vi "eventMode.vi"() -> ()   [LabVIEW 2019]
uses:
  TypeDefs/pixArrSmol.ctl
  <vilib>/Math Plots/3D Math Plots/3D Surface/3D Surface XCtrl/3D Surface.xctl
  <vilib>/Utility/error.llb/whitespace.ctl
  <vilib>/Instr/_visa.llb/VISA Flush IO Buffer Mask.ctl
  <vilib>/Utility/file.llb/Read Delimited Spreadsheet (string).vi
  <vilib>/Math Plots/3D Math Plots/3D Surface/3D Surface Datatype/Public/Plot Helper (Vector).vi
  <vilib>/Instr/_visa.llb/VISA Configure Serial Port (Instr).vi
  TypeDefs/serialSettings_Global.vi
  <vilib>/Analysis/NI_AALBase.lvlib
  <vilib>/Math Plots/3D Math Plots/3D Surface/3D Surface Datatype/3D Surface Datatype.lvclass
panel:
  out "read buffer":string
  out "Noisy Pixel List":i32[][](array[numeric])
  out "all rows":string[][](array[string])
  in  "Open CSV":bool
  out "Intensity Graph":u32[][](graph)
  out "States Out":string
  out "Current Time":timestamp
  in  "Iteration Limit":u32=4999
  out "Detector Surface":refnum<class "3D Plot Datatype.lvclass">[](xcontrol)
  out "Event Count Histogram":T1(graph)
  in  "Set emulate":bool
  out "Emulator 1":bool
  in  "Emulate?":bool
  out "Emulator 2":bool
  out "CZT 2 \nFrequency":u8 format="%d Mhz"
  in  "Set Clock":bool
  in  "Set CZT Clock":u8(ring)=2 items=["30 Mhz"=6, "25 Mhz"=5, "20 Mhz"=4, "15 Mhz"=3, "10 Mhz"=2]
  out "CZT 1\nFrequency":u8 format="%d Mhz"
  in  "Detector Chooser":bool caption="Boolean"
  out "CZT 2 Threshold":u16 format="%u KeV"
  out "Serial Number 2":u32
  out "Serial Number":u32
  in  "Clear Serial":bool
  in  "Read Serial":bool
  in  "PixOff":bool
  in  "Stop":bool
  in  "Get All Pixel Status":bool
  in  "Test Description":string caption="(Inserted in FITS header)"
  out "CZT 1 Threshold":u16 format="%u KeV"
  in  "Set Threshold":bool
  in  "Select Threshold Value":u16(slide)=20 min=20 max=200 scale=20.0..200.0
  out "Column":u8=1
  out "Row":string="A"
  out "Pixel Matrix Status":T2=[[TRUE, TRUE, TRUE, TRUE, TRUE, TRUE, TRUE, TRUE, TRUE, TRUE, TRUE, TRUE, TRUE, TRUE, TRUE, TRUE, TRUE], [TRUE, TRUE, TRUE, TRUE, TRUE, TRUE, TRUE, TRUE, TRUE, TRUE, TRUE, TRUE, TRUE, TRUE, TRUE, TRUE, TRUE], [TRUE, TRUE, TRUE, TRUE, TRUE, TRUE, TRUE, TRUE, TRUE, TRUE, TRUE, TRUE, TRUE, TRUE, TRUE, TRUE, TRUE], [TRUE, TRUE, TRUE, TRUE, TRUE, TRUE, TRUE, TRUE, TRUE, TRUE, TRUE, TRUE, TRUE, TRUE, TRUE, TRUE, TRUE], [TRUE, TRUE, TRUE, TRUE, TRUE, TRUE, TRUE, TRUE, TRUE, TRUE, TRUE, TRUE, TRUE, TRUE, TRUE, TRUE, TRUE], [TRUE, TRUE, TRUE, TRUE, TRUE, TRUE, TRUE, TRUE, TRUE, TRUE, TRUE, TRUE, TRUE, TRUE, TRUE, TRUE, TRUE], [TRUE, TRUE, TRUE, TRUE, TRUE, TRUE, TRUE, TRUE, TRUE, TRUE, TRUE, TRUE, TRUE, TRUE, TRUE, TRUE, TRUE], [TRUE, TRUE, TRUE, TRUE, TRUE, TRUE, TRUE, TRUE, TRUE, TRUE, TRUE, TRUE, TRUE, TRUE, TRUE, TRUE, TRUE], [TRUE, TRUE, TRUE, TRUE, TRUE, TRUE, TRUE, TRUE, TRUE, TRUE, TRUE, TRUE, TRUE, TRUE, TRUE, TRUE, TRUE], [TRUE, TRUE, TRUE, TRUE, TRUE, TRUE, TRUE, TRUE, TRUE, TRUE, TRUE, TRUE, TRUE, TRUE, TRUE, TRUE, TRUE], [TRUE, TRUE, TRUE, TRUE, TRUE, TRUE, TRUE, TRUE, TRUE, TRUE, TRUE, TRUE, TRUE, TRUE, TRUE, TRUE, TRUE], [TRUE, TRUE, TRUE, TRUE, TRUE, TRUE, TRUE, TRUE, TRUE, TRUE, TRUE, TRUE, TRUE, TRUE, TRUE, TRUE, TRUE], [TRUE, TRUE, TRUE, TRUE, TRUE, TRUE, TRUE, TRUE, TRUE, TRUE, TRUE, TRUE, TRUE, TRUE, TRUE, TRUE, TRUE], [TRUE, TRUE, TRUE, TRUE, TRUE, TRUE, TRUE, TRUE, TRUE, TRUE, TRUE, TRUE, TRUE, TRUE, TRUE, TRUE, TRUE], [TRUE, TRUE, TRUE, TRUE, TRUE, TRUE, TRUE, TRUE, TRUE, TRUE, TRUE, TRUE, TRUE, TRUE, TRUE, TRUE, TRUE], [TRUE, TRUE, TRUE, TRUE, TRUE, TRUE, TRUE, TRUE, TRUE, TRUE, TRUE, TRUE, TRUE, TRUE, TRUE, TRUE, TRUE]]
  in  "PixOn":bool
  in  "Choose Pixel To Toggle":u8 format="%02.0f"
  in  "Stop":bool
  in  "Start":bool
  in  "Short Description":string caption="(Appended to file name)"
  in  "User Name":string
  in  "Acquisition Period":T3={"Hours"=0, "Minutes"=0, "Seconds"=10}
  out "Event Mode":bool
  out "Iteration Count":u32
  out "FITS File Generated?":bool
  out "Time elapsed":dbl format="%<%H:%M:%S>t"
  in  "Exit":bool
  # "Pixel Matrix Settings"
  # "Event Mode Test"
  # "Event Start:    A0FF55\nEvent Stop:    A00055\nEmu +Eve :    A1FF55\nThresh Set:    EXXX55\nToggle Pixel: D0XX55\nChck All Pix: DFXX55\nRead Serial:   BXXX55\nClock Set:      C00X55"
  # "Need to add stop event mode command in LV state machine!"
  # "Energy Threshold Settings"
  # "KeV"
  # "Channel"
  # "Counts"
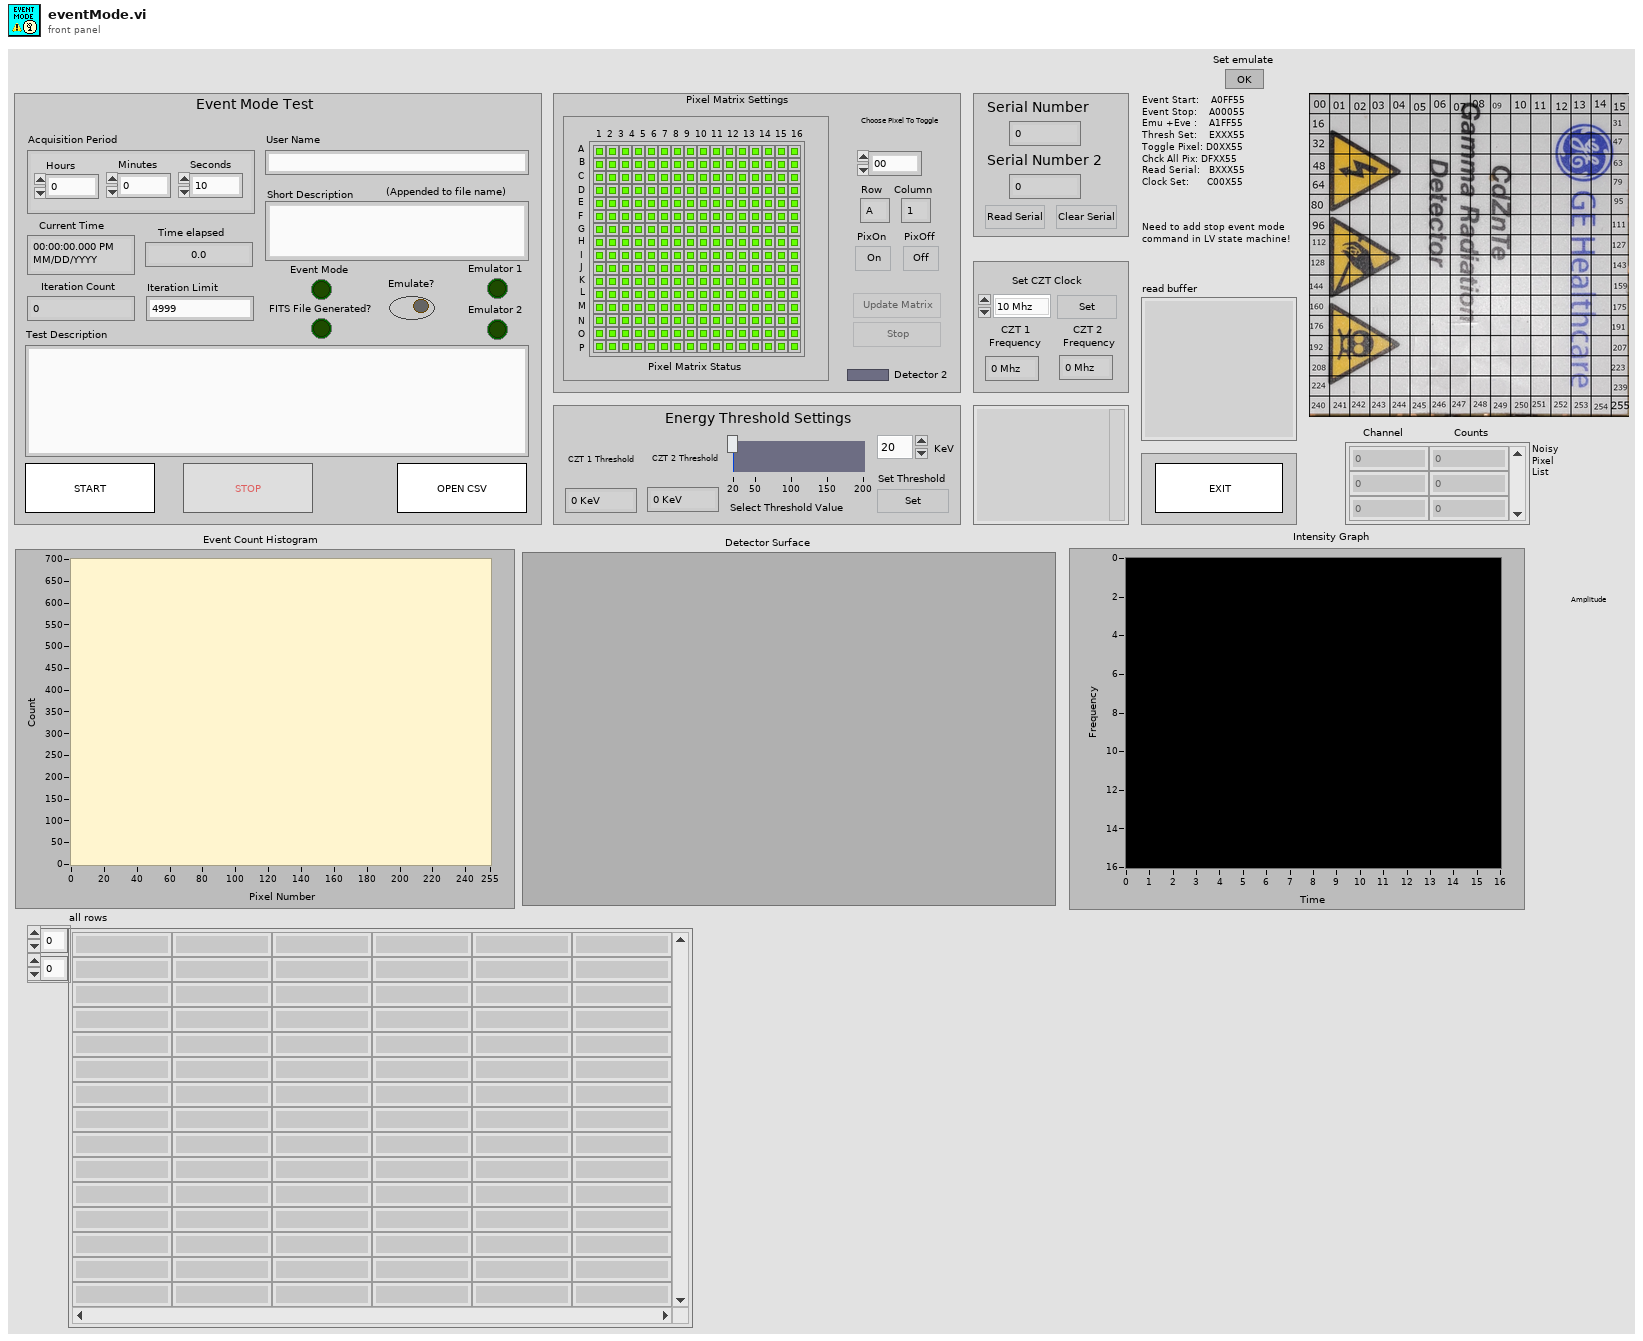
[diagram p1: front panel]
types:
  T1 = cluster{"X Values":dbl[], "Histogram: h(x)":i32[]}
  T2 = typedef "pixArrSmol.ctl" = bool[][]
  T3 = cluster{"Hours":u32, "Minutes":u32, "Seconds":u32}
  T4 = enum32{"Invalid", "Standard", "Closed", "Hidden", "Minimized", "Maximized"}
  T5 = enum32{"invalid app kind", "Development System", "Run Time System", "Student Edition", "Embedded LabVIEW", "Evaluation", "Custom"}
  T6 = enum8{"Enabled", "Disabled", "Disabled and Grayed Out"}
  T7 = cluster{"VISA resource name":refnum<visa-resource-name>, "baud rate":u32, "data bits":u16, "parity":enum16{"None", "Odd", "Even", "Mark", "Space"}, "stop bits":u16, "flow control":u16}
  T8 = cluster{"Core":cluster{"Current VI Reference":refnum<vi>, "Close Panel on Exit?":bool}, "Stop Pressed?":bool, "Start Time":dbl, "Acquisition Period":dbl, "Iteration Count":u32, "CSV File Data":cluster{"Dump txt file path":path, "Data Buffer":string, "Valid Data in Buffer":i32, "CSV file path":path, "Fits File name":string, "Test Start time":timestamp}, "User & Config Data":cluster{"User Name":string, "Short Description":string, "Description":string, "Current Threshold Value":u16}, "Pixel Status":cluster{"Pixel Number":u16, "Pixel En/Dis?":bool, "Pixel Array":bool[][], "Disabled Pixels":u8[]}}
  T9 = cluster{"Pixel Number":u16, "Pixel En/Dis?":bool, "Pixel Array":bool[][], "Disabled Pixels":u8[]}
  T10 = cluster{"User Name":string, "Short Description":string, "Description":string, "Current Threshold Value":u16}
  T11 = cluster{"Dump txt file path":path, "Data Buffer":string, "Valid Data in Buffer":i32, "CSV file path":path, "Fits File name":string, "Test Start time":timestamp}
  T12 = cluster{"Current VI Reference":refnum<vi>, "Close Panel on Exit?":bool}
  T13 = cluster{"User Name":string, "Short Description ":string, "Test Description":string, "Value":u16}
  T14 = cluster{"Dump txt file path":path, "Data buffer OUT":string, "Valid Data Buf OUT":i32, "CSV file path":path, "Fits File name":string, "Test Start time":timestamp}
  T15 = cluster{"Fits File name":string, "User Name":string, "Short Description":string, "Description":string, "Test Start time":timestamp, "Acquisition Period":dbl, "Current Threshold Value":u16, "Disabled Pixels":u8[]}
  T16 = typedef "whitespace.ctl" = u16
  T17 = typedef "VISA Flush IO Buffer Mask.ctl" = u16
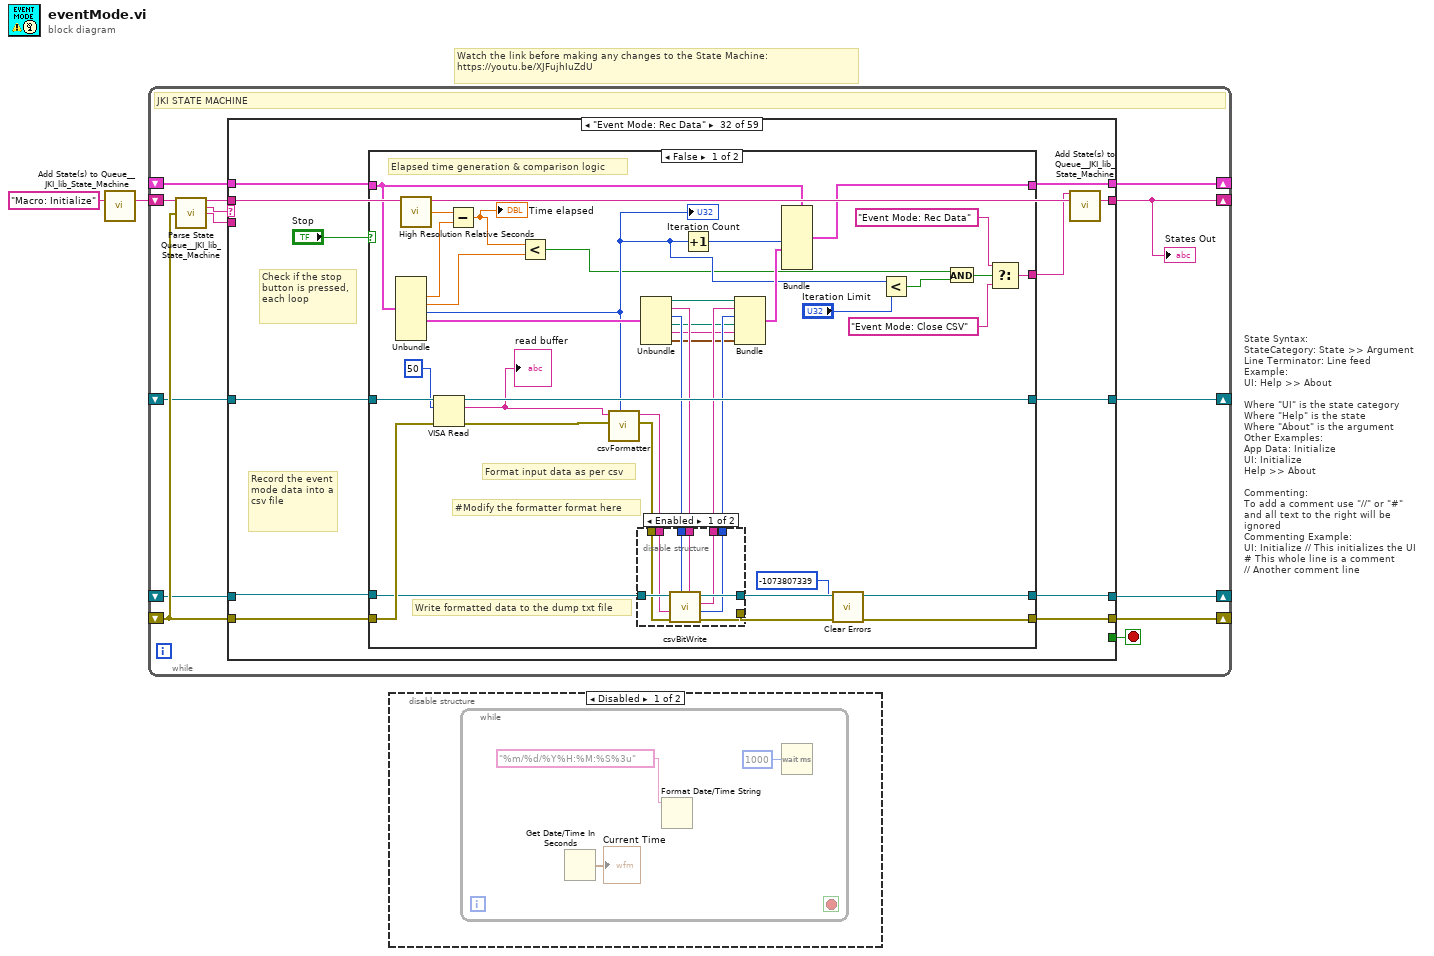
[diagram p0: block diagram]
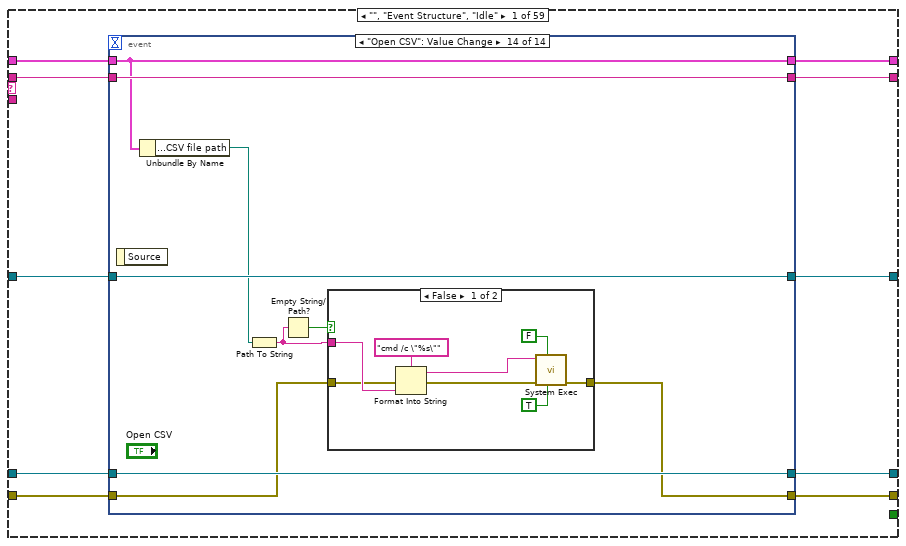
[diagram p3: hidden frame]
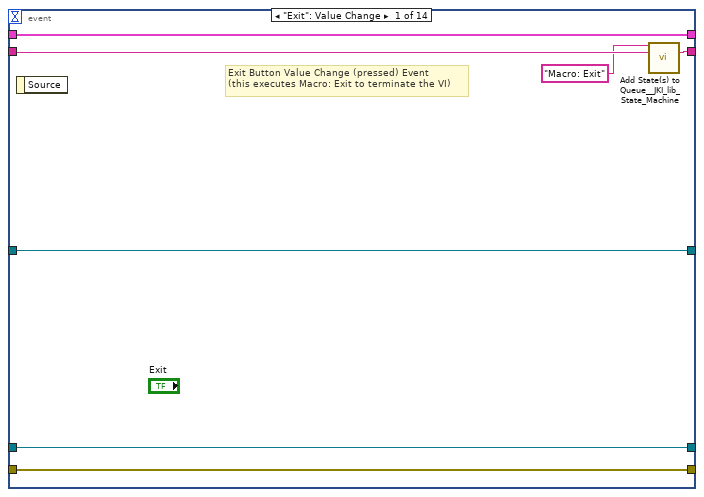
[diagram p4: hidden frame]
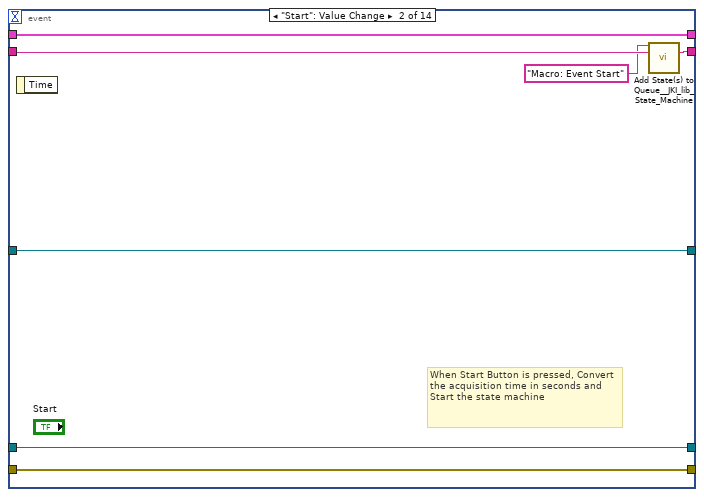
[diagram p5: hidden frame]
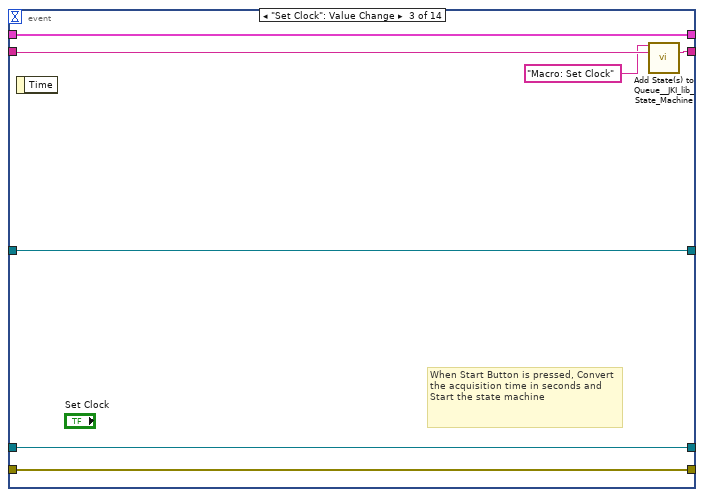
[diagram p6: hidden frame]
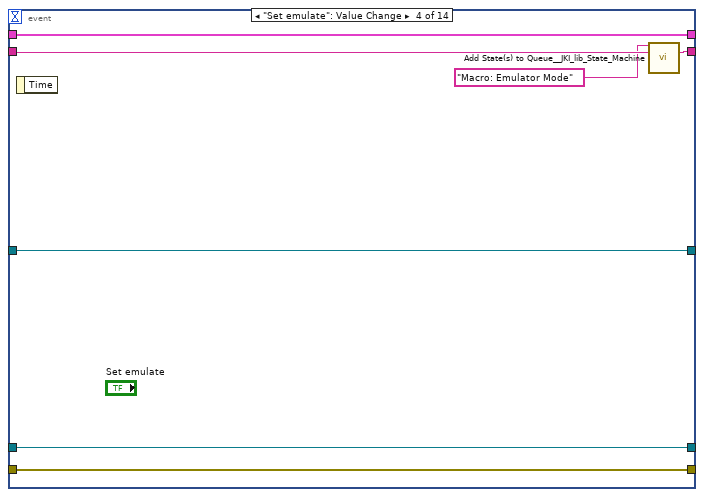
[diagram p7: hidden frame]
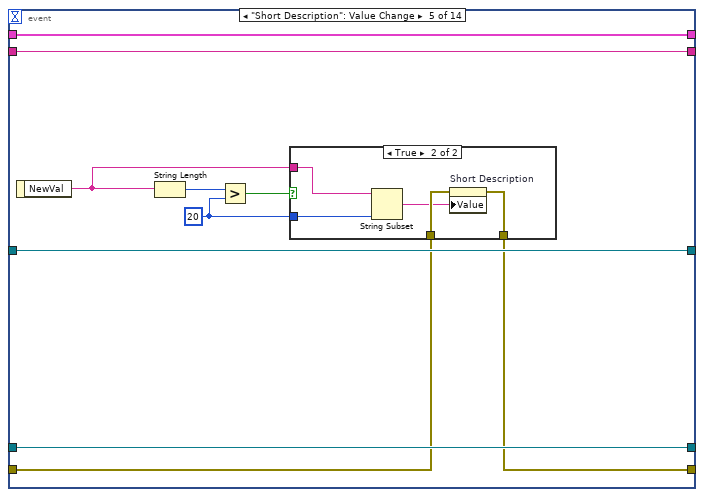
[diagram p8: hidden frame]
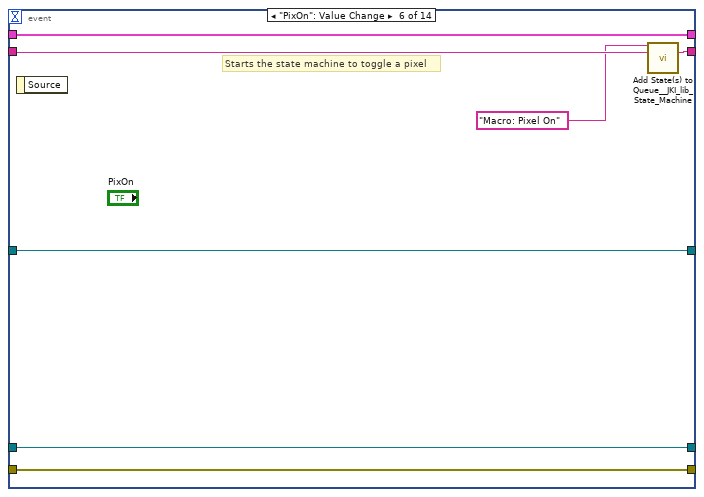
[diagram p10: hidden frame]
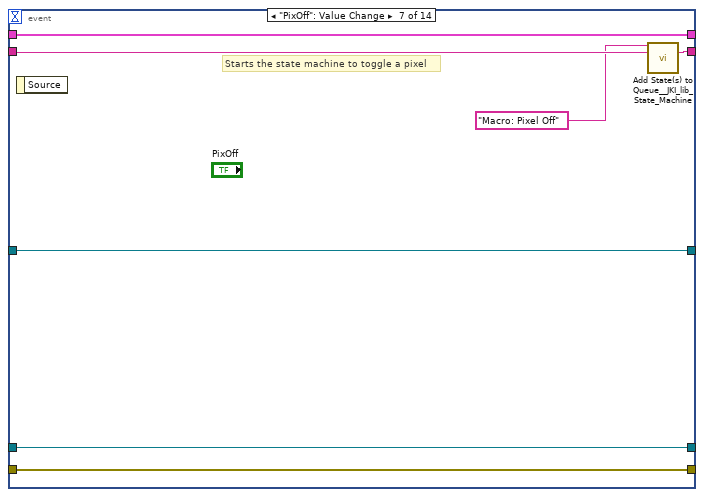
[diagram p11: hidden frame]
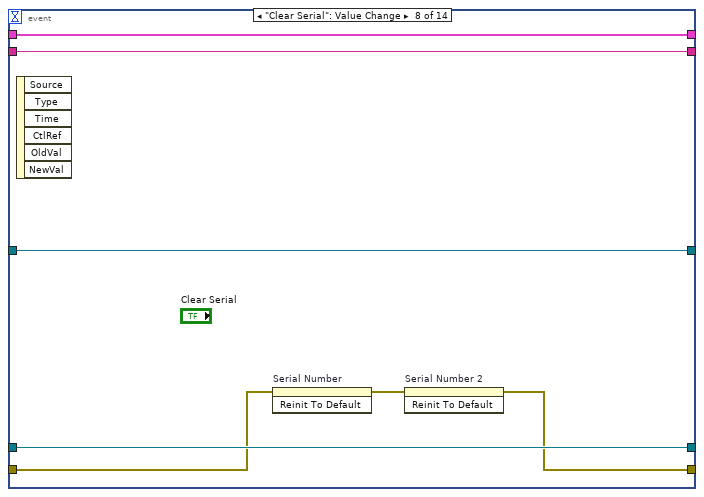
[diagram p12: hidden frame]
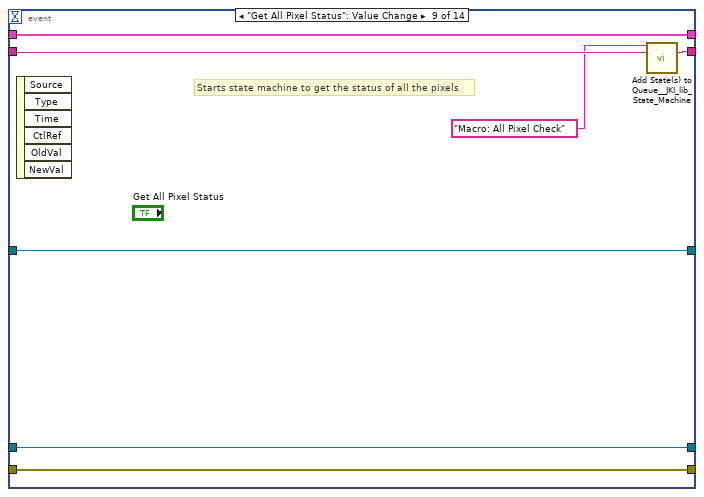
[diagram p13: hidden frame]
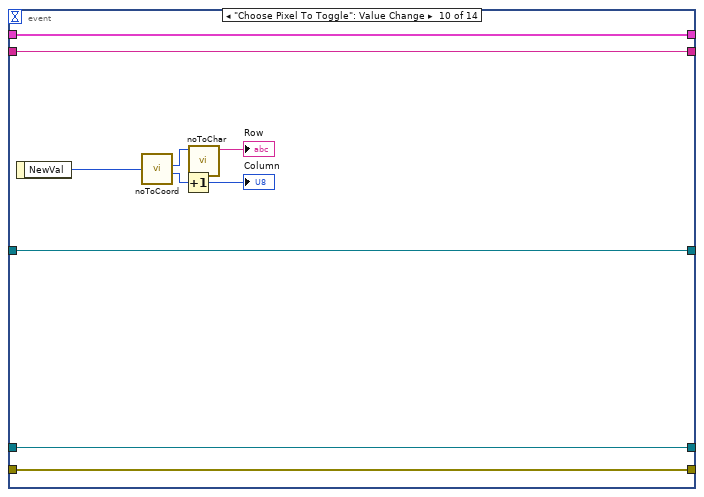
[diagram p14: hidden frame]
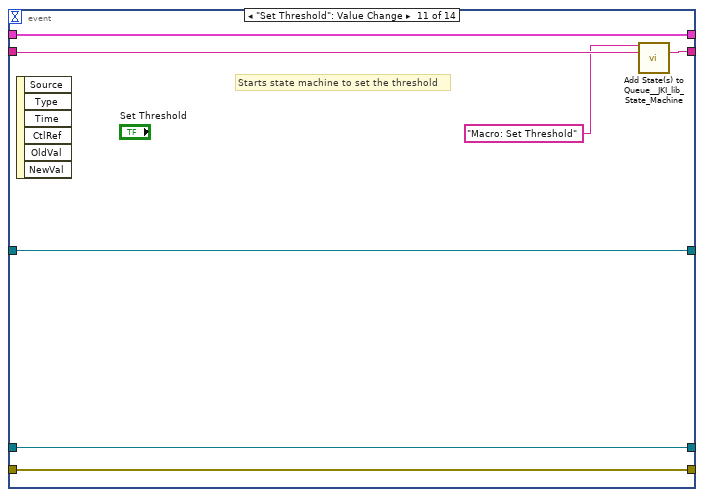
[diagram p15: hidden frame]
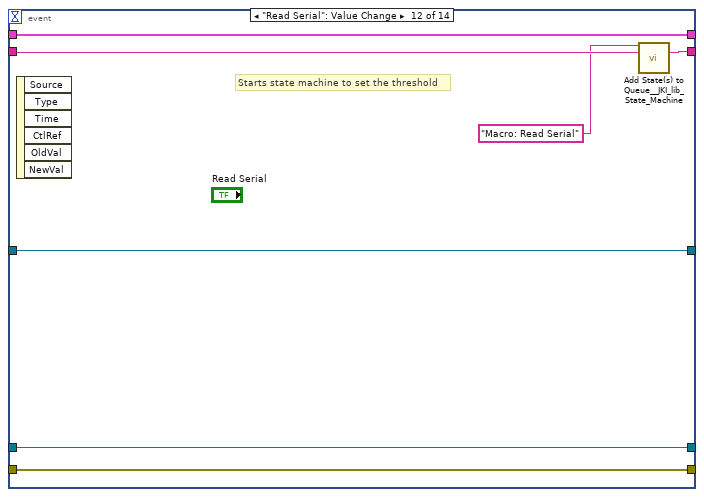
[diagram p16: hidden frame]
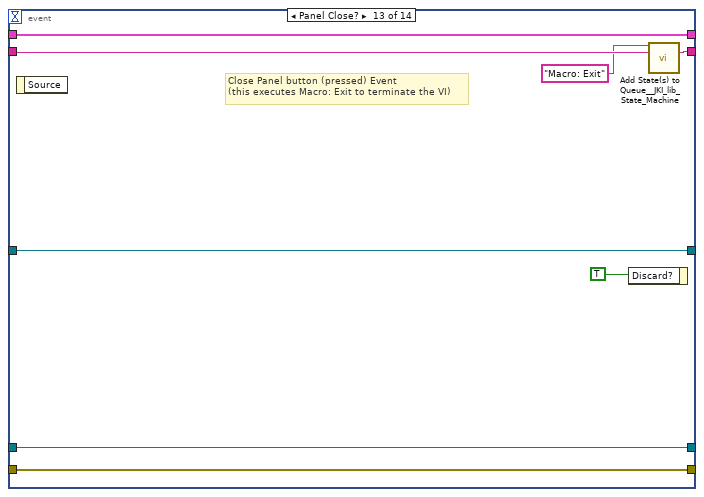
[diagram p17: hidden frame]
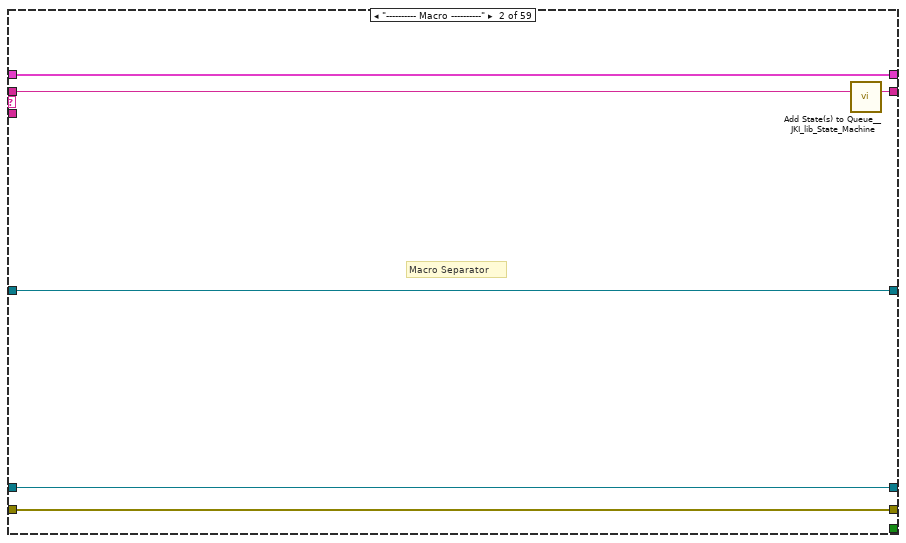
[diagram p19: hidden frame]
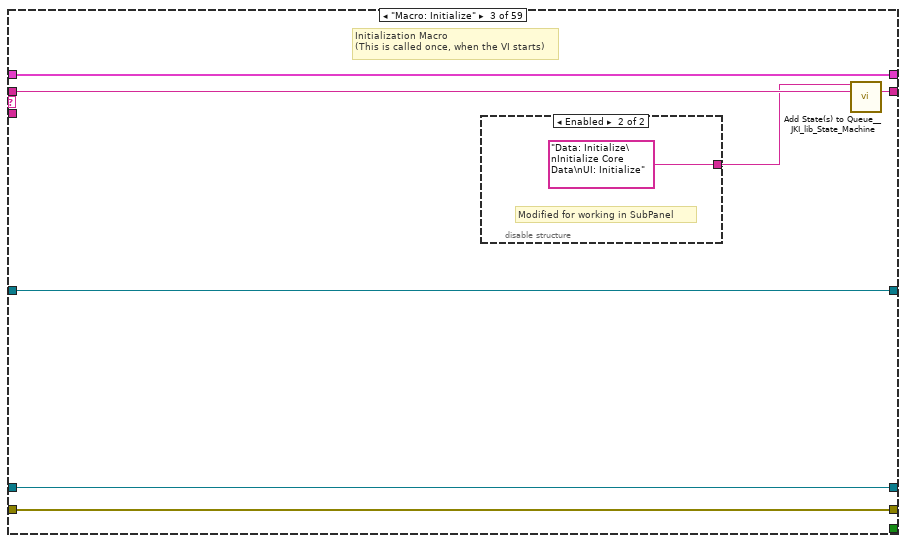
[diagram p20: hidden frame]
diagram:
  # "Watch the link before making any changes to the State Machine:\nhttps://youtu.be/XJFujhIuZdU"
  # "State Syntax:\nStateCategory: State >> Argument\nLine Terminator: Line feed\nExample:\nUI: Help >> About\n\nWhere \"UI\" is the state category\nWhere \"Help\" is the state\nWhere \"About\" is the argument\nOther Examples:\nApp Data: Initialize\nUI: Initialize\nHelp >> About\n\nCommenting:\nTo add a comment use \"//\" or \"#\" and all text to the right will be ignored\nCommenting Example:\nUI: Initialize // This initializes the UI\n# This whole line is a comment\n// Another comment line"
  n1 = call <vilib>:"Add State(s) to Queue__JKI_lib_State_Machine.vi"("State(s) in (\"\")"="Macro: Initialize") -> ("States Out"=w2:string)  [unwired: 14 in]
  n2 = while "JKI State Machine 2018" {
    shift-right: [w10] -> _
    shift-left: _ -> [w9]
    shift-right: [w12] -> _
    shift-left: _ -> [w8]
    shift-right: [w11] -> _
    shift-left: w2 -> [w13]
    shift-right: [w7] -> _
    shift-left: _ -> [w6]
    shift-right: [w5] -> _
    shift-left: _ -> [w4]
    stop <- w3 stop-if-true
    # "JKI STATE MACHINE"
    n3 = call <vilib>:"Parse State Queue__JKI_lib_State_Machine.vi"("State Queue"=w13, "Error In (no error)"=w8) -> ("Remaining States"=w15:string, "Current State"=w16:string, "Arguments"=w14:string)  [unwired: 11 in]
    n4 = case shown="\"Event Mode: Rec Data\"" w16 {
      selector: w16 -> [_ _ _ _ _ _ _ _ _ _ _ _ _ w240 _ _ _ _ _ _ _ _ _ _ _ _ _ _ _ _ _ _ _ _ _ _ _ _ _ _ _ _ _ _ _ _ _ _ _ _ _ _ _ _ _ _ _ _ _]
      tunnel: w15 -> [w26 w154 w161 w170 w177 w184 w191 w198 w205 w212 w219 w231 w237 w244 w265 _ w285 w291 w297 w303 w317 w325 w331 w365 w373 w386 w457 w474 w494 w502 w522 w572 w662 w699 w725 w731 w747 w764 w792 w807 w813 w822 w837 w874 w880 w893 w914 w920 w933 w952 w967 w980 w1005 w1011 w1027 w1056 w1062 w1082 w1099]
      tunnel: w14 -> [_ _ _ _ _ _ _ _ _ _ _ _ _ _ _ _ _ _ _ _ _ _ _ _ w368 w380 _ _ _ _ _ _ _ _ _ _ _ _ _ _ _ _ _ _ _ _ w904 _ _ w944 _ _ w995 _ _ w1046 _ w1068 w1086]
      tunnel: w9 -> [w24 w151 w158 w167 w174 w181 w188 w195 w202 w209 w216 w228 w234 w242 w258 w276 w283 w288 w294 w300 _ w320 w328 w363 w371 w382 w454 w465 w480 w508 w515 w562 w651 w696 w711 w728 w745 w762 w785 w799 w810 w820 w825 w864 w877 w891 w912 w917 w931 w950 w964 w978 w1003 w1008 w1025 w1054 w1059 w1080 w1097]
      tunnel: [w23 w152 w159 w168 w175 w182 w189 w196 w203 w210 w217 w229 w235 w246 w262 errorcluster {"status"=FALSE, "code"=0, "source"=""} ("error out") w282 w289 w295 w301 w314 w321 w329 w337 w369 w383 w455 w460 w477 w497 w514 w566 w640 w677 w706 w729 w734 w748 w770 w805 w811 w815 w828 w862 w878 w886 w900 w918 w928 w943 w965 w975 w998 w1009 w1022 w1049 w1060 w1066 w1087] -> w12
      tunnel: w8 -> [w22 w152 w159 w168 w175 w182 w189 w196 w203 w210 w217 w229 w235 w245 w262 w275 w282 w289 w295 w301 w314 w322 w329 w350 w370 w384 w455 w463 w483 w509 w513 w568 w643 w681 w707 w729 w733 w752 w787 w805 w811 w816 w832 w861 w878 w882 w908 w918 w926 w942 w965 w970 w999 w1009 w1018 w1050 w1060 w1079 w1093]
      tunnel: [w25 w153 w160 w169 w176 w183 w190 w197 w204 w211 w218 w230 w236 w243 w264 w278 w284 w290 w296 w302 w316 w324 w330 w364 w372 w385 w456 w473 w493 w510 w521 w571 w661 w698 w724 w730 w746 w763 w791 w806 w812 w821 w836 w873 w879 w892 w913 w919 w932 w951 w966 w979 w1004 w1010 w1026 w1055 w1061 w1081 w1098] -> w11
      tunnel: [_ _ _ _ _ _ _ _ _ _ _ _ _ _ _ _ TRUE _ _ _ _ _ _ _ _ _ _ _ _ _ _ _ _ _ _ _ _ _ _ _ _ _ _ _ _ _ _ _ _ _ _ _ _ _ _ _ _ _ _] -> w3
      tunnel: [w21 w151 w158 w167 w174 w181 w188 w195 w202 w209 w216 w228 w234 w242 w263 w276 w283 w288 w294 w300 w315 w320 w328 w363 w371 w382 w454 w464 w479 w508 w518 w563 w650 w696 w711 w728 w745 w762 w786 w794 w810 w820 w824 w863 w877 w891 w912 w917 w931 w950 w964 w978 w1003 w1008 w1025 w1054 w1059 w1080 w1097] -> w10
      tunnel: [w17 w149 w155 w164 w172 w179 w186 w192 w199 w206 w214 w220 w232 w238 w251 w273 w279 w286 w292 w298 w305 w318 w326 w359 w366 w378 w452 w459 w478 w501 w519 w567 w642 w694 w722 w726 w737 w755 w788 w803 w808 w817 w834 w871 w875 w888 w909 w915 w929 w947 w962 w976 w1000 w1006 w1023 w1051 w1057 w1067 _] -> w7
      tunnel: w6 -> [w18 w149 w155 w164 w172 w179 w186 w192 w199 w206 w214 w220 w232 w238 w251 w273 w279 w286 w292 w298 w305 w318 w326 w359 w366 w378 w452 w459 w478 w501 w520 w569 w644 w694 w722 w726 w743 w760 w789 w803 w808 w818 w833 w871 w875 w881 w910 w915 w927 w948 w962 w972 w1001 w1006 w1019 w1052 w1057 _ w1095]
      tunnel: [w19 w150 w156 w166 w173 w180 w187 w194 w201 w208 w215 w221 w233 w239 w252 w274 w280 w287 w293 w299 w310 w319 w327 w362 w367 w379 w453 w472 w492 w507 w516 w564 _ w697 w723 w727 w744 w761 w790 w804 w809 w819 w835 w872 w876 w890 w911 w916 w930 w949 w963 w977 w1002 w1007 w1024 w1053 w1058 w1069 w1096] -> w5
      tunnel: w4 -> [w20 w150 w156 w166 w173 w180 w187 w194 w201 w208 w215 w221 w233 w239 w252 w274 w280 w287 w293 w299 w310 w319 w327 w362 w367 w379 w453 w472 w492 w507 _ w565 w659 w697 w723 w727 w744 w761 w790 w804 w809 w819 w835 w872 w876 w890 w911 w916 w930 w949 w963 w977 w1002 w1007 w1024 w1053 w1058 w1069 w1096]
      frame "", "Event Structure", "Idle" {
        n5 = event shown="[13] \"Open CSV\": Value Change" {
          selector: _ -> [_ _ _ _ _ _ _ _ _ _ _ _ _ _]
          dyn-events: _ -> [_ _ _ _ _ _ _ _ _ _ _ _ _ _]
          timeout: _ -> [_ _ _ _ _ _ _ _ _ _ _ _ _ _]
          tunnel: w26 -> [w33 w40 w47 w54 w61 w74 w81 w88 w96 w106 w113 w120 w130 w137]
          tunnel: [w32 w39 w46 w53 w61 w75 w82 w88 w95 w106 w112 w119 w129 w137] -> w25
          tunnel: w24 -> [w31 w36 w43 w50 w62 w76 w83 w89 w97 w107 w114 w121 w127 w136]
          tunnel: [w27 w35 w42 w49 w59 w73 w80 w85 w94 w105 w111 w118 w128 w134] -> w23
          tunnel: w22 -> [w27 w35 w42 w49 w60 w73 w80 w87 w94 w105 w111 w118 w128 w133]
          tunnel: [w31 w36 w43 w50 w62 w76 w83 w89 w97 w107 w114 w121 w127 w136] -> w21
          tunnel: [w29 w37 w44 w51 w64 w77 w84 w91 w98 w108 w115 w122 w124 w139] -> w19
          tunnel: w20 -> [w29 w37 w44 w51 w64 w77 w84 w91 w98 w108 w115 w122 w124 w139]
          tunnel: w18 -> [w28 w34 w41 w48 w63 w71 w78 w90 w92 w99 w109 w116 w123 w138]
          tunnel: [w28 w34 w41 w48 w63 w71 w78 w90 w92 w99 w109 w116 w123 w138] -> w17
          event "Exit": Value Change {
            # "Exit Button Value Change (pressed) Event\n(this executes Macro: Exit to terminate the VI)"
            n6 = event-data() -> ()  [unwired: 1 in, 1 out]
            n7 = call <vilib>:"Add State(s) to Queue__JKI_lib_State_Machine.vi"("State(s) in Front (\"\")"="Macro: Exit", "State(s) in (\"\")"=w33) -> ("States Out"=w32:string)  [unwired: 13 in]
          }
          event "Start": Value Change {
            # "When Start Button is pressed, Convert the acquisition time in seconds and Start the state machine"
            n8 = event-data() -> ()  [unwired: 1 in, 1 out]
            n9 = call <vilib>:"Add State(s) to Queue__JKI_lib_State_Machine.vi"("State(s) in Front (\"\")"="Macro: Event Start", "State(s) in (\"\")"=w40) -> ("States Out"=w39:string)  [unwired: 13 in]
          }
          event "Set Clock": Value Change {
            # "When Start Button is pressed, Convert the acquisition time in seconds and Start the state machine"
            n10 = event-data() -> ()  [unwired: 1 in, 1 out]
            n11 = call <vilib>:"Add State(s) to Queue__JKI_lib_State_Machine.vi"("State(s) in Front (\"\")"="Macro: Set Clock", "State(s) in (\"\")"=w47) -> ("States Out"=w46:string)  [unwired: 13 in]
          }
          event "Set emulate": Value Change {
            n12 = event-data() -> ()  [unwired: 1 in, 1 out]
            n13 = call <vilib>:"Add State(s) to Queue__JKI_lib_State_Machine.vi"("State(s) in Front (\"\")"="Macro: Emulator Mode", "State(s) in (\"\")"=w54) -> ("States Out"=w53:string)  [unwired: 13 in]
          }
          event "Short Description": Value Change {
            w55 = 20
            n14 = event-data() -> ("NewVal"=w58:string)  [unwired: 1 in]
            n15 = String Length(string=w58) -> (length=w57:i32)
            n16 = Greater?(x=w57, y=w55) -> (0:w56:bool)
            n17 = case shown="True" w56 {
              tunnel: w60 -> [w65 w70]
              tunnel: [w65 w69] -> w59
              tunnel: w58 -> [_ w68]
              tunnel: w55 -> [_ w66]
              frame False {
              }
              frame True {
                n18 = String Subset(string=w68, length (rest)=w66) -> (substring=w67:string)  [unwired: 1 in]
                n19 = property on="Short Description" class="Str"(error in=w70, "Value"=w67) -> (error out=w69:errorcluster)  [unwired: 1 in, 1 out]
              }
            }
          }
          event "PixOn": Value Change {
            # "Starts the state machine to toggle a pixel"
            n20 = event-data() -> ()  [unwired: 1 in, 1 out]
            n21 = call <vilib>:"Add State(s) to Queue__JKI_lib_State_Machine.vi"("State(s) in Front (\"\")"="Macro: Pixel On" ("State(s) in Front (\"\")"), "State(s) in (\"\")"=w74) -> ("States Out"=w75:string)  [unwired: 13 in]
          }
          event "PixOff": Value Change {
            # "Starts the state machine to toggle a pixel"
            n22 = event-data() -> ()  [unwired: 1 in, 1 out]
            n23 = call <vilib>:"Add State(s) to Queue__JKI_lib_State_Machine.vi"("State(s) in Front (\"\")"="Macro: Pixel Off" ("State(s) in Front (\"\")"), "State(s) in (\"\")"=w81) -> ("States Out"=w82:string)  [unwired: 13 in]
          }
          event "Clear Serial": Value Change {
            n24 = event-data() -> ()  [unwired: 1 in, 6 out]
            n25 = invoke on="Serial Number" class="DigNum (strict)" method="Reinit To Default"(error in=w87) -> (error out=w86:errorcluster)  [unwired: 2 in, 2 out]
            n26 = invoke on="Serial Number 2" class="DigNum (strict)" method="Reinit To Default"(error in=w86) -> (error out=w85:errorcluster)  [unwired: 2 in, 2 out]
          }
          event "Get All Pixel Status": Value Change {
            # "Starts state machine to get the status of all the pixels"
            n27 = event-data() -> ()  [unwired: 1 in, 6 out]
            n28 = call <vilib>:"Add State(s) to Queue__JKI_lib_State_Machine.vi"("State(s) in Front (\"\")"="Macro: All Pixel Check" ("State(s) in Front (\"\")"), "State(s) in (\"\")"=w96) -> ("States Out"=w95:string)  [unwired: 13 in]
          }
          event "Choose Pixel To Toggle": Value Change {
            n29 = event-data() -> ("NewVal"=w104:u8)  [unwired: 1 in]
            n30 = call "noToCoord.vi"("Pixel number"=w104) -> ("i"=w101:u8, "j"=w103:u8)  [unwired: 6 in]
            n31 = Increment(x=w103) -> (x+1=→"Column":u8)
            n32 = call "noToChar.vi"("i"=w101) -> ("String"=→"Row":string)  [unwired: 10 in]
          }
          event "Set Threshold": Value Change {
            # "Starts state machine to set the threshold"
            n33 = event-data() -> ()  [unwired: 1 in, 6 out]
            n34 = call <vilib>:"Add State(s) to Queue__JKI_lib_State_Machine.vi"("State(s) in Front (\"\")"="Macro: Set Threshold" ("State(s) in Front (\"\")"), "State(s) in (\"\")"=w113) -> ("States Out"=w112:string)  [unwired: 13 in]
          }
          event "Read Serial": Value Change {
            # "Starts state machine to set the threshold"
            n35 = event-data() -> ()  [unwired: 1 in, 6 out]
            n36 = call <vilib>:"Add State(s) to Queue__JKI_lib_State_Machine.vi"("State(s) in Front (\"\")"="Macro: Read Serial" ("State(s) in Front (\"\")"), "State(s) in (\"\")"=w120) -> ("States Out"=w119:string)  [unwired: 13 in]
          }
          event Panel Close? {
            # "Close Panel button (pressed) Event\n(this executes Macro: Exit to terminate the VI)"
            n37 = event-data() -> ()  [unwired: 1 in, 1 out]
            n38 = event-data("Discard?"=TRUE) -> ()  [unwired: 1 in, 1 out]
            n39 = call <vilib>:"Add State(s) to Queue__JKI_lib_State_Machine.vi"("State(s) in Front (\"\")"="Macro: Exit", "State(s) in (\"\")"=w130) -> ("States Out"=w129:string)  [unwired: 13 in]
          }
          event "Open CSV": Value Change {
            n40 = event-data() -> ()  [unwired: 1 in, 1 out]
            n41 = Unbundle By Name(w136) -> ("CSV File Data.CSV file path"=w135:path)
            n42 = Path To String(path=w135) -> (string=w132:string)
            n43 = Empty String/Path?(string/path=w132) -> (empty?=w131:bool)
            n44 = case shown="False" w131 {
              tunnel: w132 -> [w147 _]
              tunnel: [w141 w148] -> w134
              tunnel: w133 -> [w140 w148]
              frame False {
                n45 = Format Into String(format string="cmd /c \"%s\"", error in=w140, w147) -> (resulting string=w145:string, error out=w146:errorcluster)  [unwired: 1 in]
                n46 = call <vilib>:"System Exec.vi"("run minimized? (F)"=TRUE ("run minimized?"), "wait until completion? (T)"=FALSE ("wait until completion?"), "error in (no error)"=w146, "command line"=w145) -> ("error out"=w141:errorcluster)  [unwired: 4 in, 3 out]
              }
              frame True {
              }
            }
          }
        }
      }
      frame "---------- Macro ----------" {
        # "Macro Separator"
        n47 = call <vilib>:"Add State(s) to Queue__JKI_lib_State_Machine.vi"("State(s) in (\"\")"=w154) -> ("States Out"=w153:string)  [unwired: 14 in]
      }
      frame "Macro: Initialize" {
        # "Initialization Macro\n(This is called once, when the VI starts)"
        n48 = disable-structure shown="Enabled" {
          disable-tunnel: [w162 "Data: Initialize\nInitialize Core Data\nUI: Initialize"] -> w157
          frame Disabled {
            w162 = "Data: Initialize\nInitialize Core Data\nUI: Initialize\nUI: Front Panel State >> Standard"  # Data: Initialize Initialize Core Data UI: Initialize UI: Front Panel State >> Standard
          }
          frame Enabled {
            # "Modified for working in SubPanel"
          }
        }
        n49 = call <vilib>:"Add State(s) to Queue__JKI_lib_State_Machine.vi"("State(s) in Front (\"\")"=w157, "State(s) in (\"\")"=w161) -> ("States Out"=w160:string)  [unwired: 13 in]
      }
      frame "Macro: Event Start" {
        # "Do not put any code in this frame.\n(It is a separator no-op. You can make a copy of this frame to create a new Macro frame)"
        n50 = call <vilib>:"Add State(s) to Queue__JKI_lib_State_Machine.vi"("State(s) in Front (\"\")"="Event Mode: Data Init\nEvent Mode: Data Get\nEvent Mode: Data Verif\nUART Comm: Init >>Event Mode: Send Cmd", "State(s) in (\"\")"=w170) -> ("States Out"=w169:string)  [unwired: 13 in]
      }
      frame "Macro: Pixel On" {
        # "Do not put any code in this frame.\n(It is a separator no-op. You can make a copy of this frame to create a new Macro frame)"
        n51 = call <vilib>:"Add State(s) to Queue__JKI_lib_State_Machine.vi"("State(s) in Front (\"\")"="UART Comm: Init >>Pixel Status: Pix Send On\nPixel Status: Pix Rec\nPixel Status: Update Pix Matrix>> UART Comm: Close" ("State(s) in Front (\"\")"), "State(s) in (\"\")"=w177) -> ("States Out"=w176:string)  [unwired: 13 in]
      }
      frame "Macro: Pixel Off" {
        # "Do not put any code in this frame.\n(It is a separator no-op. You can make a copy of this frame to create a new Macro frame)"
        n52 = call <vilib>:"Add State(s) to Queue__JKI_lib_State_Machine.vi"("State(s) in Front (\"\")"="UART Comm: Init >>Pixel Status: Pix Send Off\nPixel Status: Pix Rec\nPixel Status: Update Pix Matrix>> UART Comm: Close" ("State(s) in Front (\"\")"), "State(s) in (\"\")"=w184) -> ("States Out"=w183:string)  [unwired: 13 in]
      }
      frame "Macro: All Pixel Check" {
        n53 = call <vilib>:"Add State(s) to Queue__JKI_lib_State_Machine.vi"("State(s) in Front (\"\")"="UART Comm: Init >>All Pixel Status: Pix Send All\nAll Pixel Status: Pix Rec All" ("State(s) in Front (\"\")"), "State(s) in (\"\")"=w191) -> ("States Out"=w190:string)  [unwired: 13 in]
      }
      frame "Macro: Set Threshold" {
        # "Do not put any code in this frame.\n(It is a separator no-op. You can make a copy of this frame to create a new Macro frame)"
        n54 = call <vilib>:"Add State(s) to Queue__JKI_lib_State_Machine.vi"("State(s) in Front (\"\")"="UART Comm: Init >>Threshold: Set Thresh\nThreshold: Get Thresh >> UART Comm: Close" ("State(s) in Front (\"\")"), "State(s) in (\"\")"=w198) -> ("States Out"=w197:string)  [unwired: 13 in]
      }
      frame "Macro: Emulator Mode" {
        # "Do not put any code in this frame.\n(It is a separator no-op. You can make a copy of this frame to create a new Macro frame)"
        n55 = call <vilib>:"Add State(s) to Queue__JKI_lib_State_Machine.vi"("State(s) in Front (\"\")"="UART Comm: Init >>Emulator: Set Mode\nEmulator: Get Mode>> UART Comm: Close" ("State(s) in Front (\"\")"), "State(s) in (\"\")"=w205) -> ("States Out"=w204:string)  [unwired: 13 in]
      }
      frame "Macro: Set Clock" {
        # "Do not put any code in this frame.\n(It is a separator no-op. You can make a copy of this frame to create a new Macro frame)"
        n56 = call <vilib>:"Add State(s) to Queue__JKI_lib_State_Machine.vi"("State(s) in Front (\"\")"="UART Comm: Init >>Clock: Set Clock\nClock: Get Clock>> UART Comm: Close" ("State(s) in Front (\"\")"), "State(s) in (\"\")"=w212) -> ("States Out"=w211:string)  [unwired: 13 in]
      }
      frame "Macro: Read Serial" {
        # "Do not put any code in this frame.\n(It is a separator no-op. You can make a copy of this frame to create a new Macro frame)"
        n57 = call <vilib>:"Add State(s) to Queue__JKI_lib_State_Machine.vi"("State(s) in Front (\"\")"="UART Comm: Init >>Serial Number: Send Command\nSerial Number: Get Number>>UART Comm: Close" ("State(s) in Front (\"\")"), "State(s) in (\"\")"=w219) -> ("States Out"=w218:string)  [unwired: 13 in]
      }
      frame "Macro: Exit" {
        # "Exit Macro\n(This is called once, when the VI exits)"
        n58 = Unbundle By Name(w228) -> ("Core.Close Panel on Exit?"=w227:bool)
        n59 = Select(t="UI: Front Panel State >> Close", s=w227, f="") -> (s? t:f=w224:string)
        n60 = call <vilib>:"Add State(s) to Queue__JKI_lib_State_Machine.vi"("State(s) in (\"\")"=w224, "State(s) at Back (\"\")"="Data: Cleanup\nExit") -> ("States Out"=w222:string)  [unwired: 13 in]
        n61 = call <vilib>:"Add State(s) to Queue__JKI_lib_State_Machine.vi"("State(s) in Front (\"\")"=w222, "State(s) in (\"\")"=w231) -> ("States Out"=w230:string)  [unwired: 13 in]
      }
      frame "---------- Core ----------" {
        # "Core Separator"
        n62 = call <vilib>:"Add State(s) to Queue__JKI_lib_State_Machine.vi"("State(s) in (\"\")"=w237) -> ("States Out"=w236:string)  [unwired: 14 in]
      }
      frame Default {
        w249 = 42 items=["No error", "Argument error", "Memory is full", "Out of zone", "End of file", "File already open", "Generic file I/O error", "File not found", "File permission error", "Disk is full", "Duplicate path", "Too many files open", "System feature not enabled", "Resource file not found", "Cannot add resource", "Resource not found", "Image not found", "Image memory error", "Pen does not exist", "Config type invalid", "Config token not found", "Config parse error", "Config memory error", "Bad external code format", "Bad external code offset", "External code not present", "Null window", "Destroy window error", "Null menu", "Print aborted", "Bad print record", "Print driver error", "Windows error during printing", "Memory error during printing", "Print dialog error", "Generic print error", "Invalid device refnum", "Device not found", "Device parameter error", "Device unit error", "Cannot open device", "Device call aborted", "Generic error", "Cancelled by user", "Object ID too low", "Object ID too high", "Object not in heap", "Unknown heap", "Unknown object (invalid DefProc)", "Unknown object (DefProc not in table)", "Message out of range", "Invalid (null) method", "Unknown message", "Manager call not supported", "Bad address", "Network operation in progress", "Network operation timed out", "Connection is busy", "Network attribute not supported", "Network error", "Address in use", "System out of memory", "Connection aborted", "Connection refused", "Not connected", "Already connected", "Connection closed", "Initialization error (interapplication manager)", "Bad occurrence", "Wait on unbound occurrence handler", "Occurrence queue overflow", "Datalog type conflict", "Unused", "Unrecognized type (interapplication manager)", "Memory corrupt", "Failed to make temporary DLL", "Old CIN version", "Drag socket not found", "Failed to load drop-object", "Failed to register OLE object", "Failed to release OLE object", "Format specifier type mismatch", "Unknown format specifier", "Too few format specifiers", "Too many format specifiers", "Scan failed", "Newer CIN version", "Error converting to variant", "Runtime menu error", "Password tampered", "Variant attribute not found", "Incompatible variant data type", "Event data is not available", "Event Store is not present", "Occurrence is not found", "Event Queue is not created", "Event info is not available", "Refnum passed is NULL", "Error retrieving Class GUID", "Error retrieving CoClass GUID", "Error retrieving TypeLib GUID.", "Bad built application magic bytes.", "Specific driver is different from the specific driver associated with the Logical Name.", "There is no session opened to the class driver.", "Max Error", "MAX - Error with config objects", "MAX - Error loading configuration", "MAX - Group not supported"]
        # "Current State"
        # "Do not delete, rename, or modify this frame.\n(this is used to capture unhandled states and typos)"
        # "Handle mistyped state name (developer tool)"
        n63 = Format Into String(format string="Software Exception: Unhandled State \"%s\"." ("message"), error in=w245, w240) -> (resulting string=w248:string, error out=w247:errorcluster)  [unwired: 1 in]
        n64 = call <vilib>:"Error Cluster From Error Code.vi"("show call chain? (False)"=TRUE, "error in (no error)"=w247, "error message (\"\")"=w248, "error code (0)"=w249) -> ("error out"=w246:errorcluster)  [unwired: 5 in]
        n65 = call <vilib>:"Add State(s) to Queue__JKI_lib_State_Machine.vi"("State(s) in (\"\")"=w244) -> ("States Out"=w243:string)  [unwired: 14 in]
      }
      frame "Initialize Core Data" {
        # "Do not delete, rename, or modify this frame.\n(this is used to determine panel behavior on exit)"
        # "originally closed?"
        # "exe?"
        # "If panel starts closed or is an EXE, then close it when we exit"
        n66 = property class="VI"() -> ("FP.State"=w255:T4)  [unwired: 2 in, 2 out]
        n67 = property class="App"() -> ("App.Kind"=w261:T5)  [unwired: 2 in, 2 out]
        n68 = control-ref of="Current VI Reference"() -> (w256:refnum<vi>)
        n69 = Equal?(x=w255, y=T4."Closed" ("Front Panel Window:State")) -> (x = y?=w253:bool)
        n70 = Equal?(x=w261, y=T5."Run Time System" ("Application:Kind")) -> (x = y?=w259:bool)
        n71 = Or(x=w253, y=w259) -> (x .or. y?=w257:bool)
        n72 = Bundle By Name(cluster=w258, "Core.Current VI Reference"=w256, "Core.Close Panel on Exit?"=w257) -> (w263:T8)
        n73 = call <vilib>:"Add State(s) to Queue__JKI_lib_State_Machine.vi"("State(s) in (\"\")"=w265) -> ("States Out"=w264:string)  [unwired: 14 in]
      }
      frame "Error Handler" {
        # "Close the UART communication if there was a timeout error"
        # "Unhandled Error -- Display it"
        # "Handle any errors here.\nYou can also output any states to clean-up after errors occur"
        # "Clear error"
        n74 = call <vilib>:"General Error Handler.vi"("error in (no error)"=w275) -> ("error out"=w272:errorcluster)  [unwired: 10 in, 4 out]
        n75 = Unbundle(w272) -> ("code"=w269:i32)  [unwired: 2 out]
        n76 = Equal?(x=-1073807339, y=w269) -> (x = y?=w268:bool)
        n77 = Select(t="UART Comm: Close", s=w268, f="") -> (s? t:f=w267:string)
        n78 = call <vilib>:"Add State(s) to Queue__JKI_lib_State_Machine.vi"("State(s) in Front (\"\")"=w267) -> ("States Out"=w278:string)  [unwired: 14 in]
      }
      frame "Exit" {
        # "Handles the exit funcitonality"
        n79 = call <vilib>:"Add State(s) to Queue__JKI_lib_State_Machine.vi"("State(s) in (\"\")"=w285) -> ("States Out"=w284:string)  [unwired: 14 in]
      }
      frame "---------- Hardware ----------" {
        # "Hardware Separator"
        n80 = call <vilib>:"Add State(s) to Queue__JKI_lib_State_Machine.vi"("State(s) in (\"\")"=w291) -> ("States Out"=w290:string)  [unwired: 14 in]
      }
      frame "Hardware: Setup DAQ" {
        # "Hardware Separator"
        n81 = call <vilib>:"Add State(s) to Queue__JKI_lib_State_Machine.vi"("State(s) in (\"\")"=w297) -> ("States Out"=w296:string)  [unwired: 14 in]
      }
      frame "---------- Data ----------" {
        n82 = call <vilib>:"Add State(s) to Queue__JKI_lib_State_Machine.vi"("State(s) in (\"\")"=w303) -> ("States Out"=w302:string)  [unwired: 14 in]
      }
      frame "Data: Initialize" {
        w304 = T9 {"Pixel Number"=0, "Pixel En/Dis?"=FALSE, "Pixel Array"=[[TRUE, TRUE, TRUE, TRUE, TRUE, TRUE, TRUE, TRUE, TRUE, TRUE, TRUE, TRUE, TRUE, TRUE, TRUE, TRUE, TRUE], [TRUE, TRUE, TRUE, TRUE, TRUE, TRUE, TRUE, TRUE, TRUE, TRUE, TRUE, TRUE, TRUE, TRUE, TRUE, TRUE, TRUE], [TRUE, TRUE, TRUE, TRUE, TRUE, TRUE, TRUE, TRUE, TRUE, TRUE, TRUE, TRUE, TRUE, TRUE, TRUE, TRUE, TRUE], [TRUE, TRUE, TRUE, TRUE, TRUE, TRUE, TRUE, TRUE, TRUE, TRUE, TRUE, TRUE, TRUE, TRUE, TRUE, TRUE, TRUE], [TRUE, TRUE, TRUE, TRUE, TRUE, TRUE, TRUE, TRUE, TRUE, TRUE, TRUE, TRUE, TRUE, TRUE, TRUE, TRUE, TRUE], [TRUE, TRUE, TRUE, TRUE, TRUE, TRUE, TRUE, TRUE, TRUE, TRUE, TRUE, TRUE, TRUE, TRUE, TRUE, TRUE, TRUE], [TRUE, TRUE, TRUE, TRUE, TRUE, TRUE, TRUE, TRUE, TRUE, TRUE, TRUE, TRUE, TRUE, TRUE, TRUE, TRUE, TRUE], [TRUE, TRUE, TRUE, TRUE, TRUE, TRUE, TRUE, TRUE, TRUE, TRUE, TRUE, TRUE, TRUE, TRUE, TRUE, TRUE, TRUE], [TRUE, TRUE, TRUE, TRUE, TRUE, TRUE, TRUE, TRUE, TRUE, TRUE, TRUE, TRUE, TRUE, TRUE, TRUE, TRUE, TRUE], [TRUE, TRUE, TRUE, TRUE, TRUE, TRUE, TRUE, TRUE, TRUE, TRUE, TRUE, TRUE, TRUE, TRUE, TRUE, TRUE, TRUE], [TRUE, TRUE, TRUE, TRUE, TRUE, TRUE, TRUE, TRUE, TRUE, TRUE, TRUE, TRUE, TRUE, TRUE, TRUE, TRUE, TRUE], [TRUE, TRUE, TRUE, TRUE, TRUE, TRUE, TRUE, TRUE, TRUE, TRUE, TRUE, TRUE, TRUE, TRUE, TRUE, TRUE, TRUE], [TRUE, TRUE, TRUE, TRUE, TRUE, TRUE, TRUE, TRUE, TRUE, TRUE, TRUE, TRUE, TRUE, TRUE, TRUE, TRUE, TRUE], [TRUE, TRUE, TRUE, TRUE, TRUE, TRUE, TRUE, TRUE, TRUE, TRUE, TRUE, TRUE, TRUE, TRUE, TRUE, TRUE, TRUE], [TRUE, TRUE, TRUE, TRUE, TRUE, TRUE, TRUE, TRUE, TRUE, TRUE, TRUE, TRUE, TRUE, TRUE, TRUE, TRUE, TRUE], [TRUE, TRUE, TRUE, TRUE, TRUE, TRUE, TRUE, TRUE, TRUE, TRUE, TRUE, TRUE, TRUE, TRUE, TRUE, TRUE, TRUE]], "Disabled Pixels"=[]}  # Pixel Status
        w306 = T10 {"User Name"="", "Short Description"="", "Description"="", "Current Threshold Value"=0}  # User & Config Data
        w307 = T11 {"Dump txt file path"=path "", "Data Buffer"="", "Valid Data in Buffer"=0, "CSV file path"=path "", "Fits File name"="", "Test Start time"=timestamp(0 s since 1904-01-01)}  # CSV File Data
        w309 = T12 {"Current VI Reference"=refnum, "Close Panel on Exit?"=FALSE}  # Core
        w308 = u32 0  # Iteration Count
        w311 = 0.0  # Start Time
        w312 = 0.0  # Acquisition Period
        w313 = TRUE  # Stop Pressed?
        # "do not delete - used by framework"
        # "Data names and types of shift register data are defined by this bundle."
        # "Initialize the shift-register data, here.\n(data names are defined by what you wire into the bundle function)"
        n83 = Bundle("Core"=w309, "Stop Pressed?"=w313, "Start Time"=w311, "Acquisition Period"=w312, "Iteration Count"=w308, "CSV File Data"=w307, "User & Config Data"=w306, "Pixel Status"=w304) -> (w315:T8)  [unwired: 1 in]
        n84 = call <vilib>:"Add State(s) to Queue__JKI_lib_State_Machine.vi"("State(s) in (\"\")"=w317) -> ("States Out"=w316:string)  [unwired: 14 in]
      }
      frame "Data: Cleanup" {
        # "Cleanup any data and references, here.\n(this is called automatically, by the Macro: Exit)"
        n85 = Unbundle By Name(w320) -> ("Core.Current VI Reference"=w323:refnum<vi>)
        n86 = Close Reference(reference=w323, error in (no error)=w322) -> (error out=w321:errorcluster)
        n87 = call <vilib>:"Add State(s) to Queue__JKI_lib_State_Machine.vi"("State(s) in (\"\")"=w325) -> ("States Out"=w324:string)  [unwired: 14 in]
      }
      frame "---------- UI ----------" {
        # "UI Separator"
        n88 = call <vilib>:"Add State(s) to Queue__JKI_lib_State_Machine.vi"("State(s) in (\"\")"=w331) -> ("States Out"=w330:string)  [unwired: 14 in]
      }
      frame "UI: Initialize" {
        w334 = T6."Disabled and Grayed Out" ("Disabled")
        # "Initialize the User Interface, here.\n(this is called automatically, by the Macro: Init)"
        n89 = invoke on="Test Description" class="Str" method="Reinit To Default"(error in=w350) -> (error out=w352:errorcluster)  [unwired: 2 in, 2 out]
        n90 = invoke on="Select Threshold Value" class="Slide (strict)" method="Reinit To Default"(error in=w350) -> (error out=w353:errorcluster)  [unwired: 2 in, 2 out]
        n91 = invoke on="CZT 1 Threshold" class="DigNum (strict)" method="Reinit To Default"(error in=w350) -> (error out=w354:errorcluster)  [unwired: 2 in, 2 out]
        n92 = invoke on="Serial Number" class="DigNum (strict)" method="Reinit To Default"(error in=w350) -> (error out=w351:errorcluster)  [unwired: 2 in, 2 out]
        n93 = invoke on="CZT 2 Threshold" class="DigNum (strict)" method="Reinit To Default"(error in=w350) -> (error out=w349:errorcluster)  [unwired: 2 in, 2 out]
        n94 = invoke on="Column" class="DigNum (strict)" method="Reinit To Default"(error in=w351) -> (error out=w356:errorcluster)  [unwired: 2 in, 2 out]
        n95 = invoke on="Row" class="Str" method="Reinit To Default"(error in=w350) -> (error out=w357:errorcluster)  [unwired: 2 in, 2 out]
        n96 = invoke on="Pixel Matrix Status" class="Arr (strict)" method="Reinit To Default"(error in=w349) -> (error out=w358:errorcluster)  [unwired: 2 in, 2 out]
        n97 = invoke on="Event Mode" class="Bool (strict)" method="Reinit To Default"(error in=w352) -> (error out=w360:errorcluster)  [unwired: 2 in, 2 out]
        n98 = invoke on="User Name" class="Str" method="Reinit To Default"(error in=w353) -> (error out=w361:errorcluster)  [unwired: 2 in, 2 out]
        n99 = invoke on="Short Description" class="Str" method="Reinit To Default"(error in=w354) -> (error out=w355:errorcluster)  [unwired: 2 in, 2 out]
        n100 = invoke on="Choose Pixel To Toggle" class="DigNum (strict)" method="Reinit To Default"(error in=w356) -> (error out=w348:errorcluster)  [unwired: 2 in, 2 out]
        n101 = property on="Stop" class="Bool (strict)"(error in=w357, "DisabledEnum"=w334) -> (error out=w336:errorcluster)  [unwired: 1 in, 1 out]
        n102 = invoke on="FITS File Generated?" class="Bool (strict)" method="Reinit To Default"(error in=w358) -> (error out=w344:errorcluster)  [unwired: 2 in, 2 out]
        n103 = invoke on="Iteration Count" class="DigNum (strict)" method="Reinit To Default"(error in=w360) -> (error out=w345:errorcluster)  [unwired: 2 in, 2 out]
        n104 = invoke on="Time elapsed" class="DigNum (strict)" method="Reinit To Default"(error in=w361) -> (error out=w343:errorcluster)  [unwired: 2 in, 2 out]
        n105 = invoke on="Acquisition Period" class="Clust (strict)" method="Reinit To Default"(error in=w355) -> (error out=w342:errorcluster)  [unwired: 2 in, 2 out]
        n106 = property on="Open CSV" class="Bool"(error in=w336, "DisabledEnum"=w334) -> (error out=w335:errorcluster)  [unwired: 1 in, 1 out]
        n107 = invoke on="CZT 1 Frequency" class="DigNum (strict)" method="Reinit To Default"(error in=w344) -> (error out=w333:errorcluster)  [unwired: 2 in, 2 out]
        n108 = invoke on="Emulator 2" class="Bool (strict)" method="Reinit To Default"(error in=w342) -> (error out=w341:errorcluster)  [unwired: 2 in, 2 out]
        n109 = invoke on="Serial Number 2" class="DigNum (strict)" method="Reinit To Default"(error in=w348) -> (error out=w339:errorcluster)  [unwired: 2 in, 2 out]
        n110 = invoke on="Emulator 1" class="Bool (strict)" method="Reinit To Default"(error in=w343) -> (error out=w340:errorcluster)  [unwired: 2 in, 2 out]
        n111 = invoke on="CZT 2 Frequency" class="DigNum (strict)" method="Reinit To Default"(error in=w345) -> (error out=w347:errorcluster)  [unwired: 2 in, 2 out]
        n112 = invoke on="Emulate?" class="Bool (strict)" method="Reinit To Default"(error in=w339) -> (error out=w338:errorcluster)  [unwired: 2 in, 2 out]
        n113 = invoke on="Set Clock" class="Bool" method="Reinit To Default"(error in=w335) -> (error out=w346:errorcluster)  [unwired: 2 in, 2 out]
        n114 = invoke on="Noisy Pixel List" class="Arr (strict)" method="Reinit To Default"(error in=w333) -> (error out=w332:errorcluster)  [unwired: 2 in, 2 out]
        n115 = Merge Errors(w338, w346, w332, w347, w340, w341) -> (w337:errorcluster)
        n116 = call <vilib>:"Add State(s) to Queue__JKI_lib_State_Machine.vi"("State(s) in (\"\")"=w365) -> ("States Out"=w364:string)  [unwired: 14 in]
      }
      frame "UI: Cursor Set" {
        # "Argument"
        # "Set and Unset Cursor Busy.\n(Usage: \"UI: Cursor Set >> Busy|Idle\")"
        n117 = case shown="\"Idle\", Default" w368 {
          tunnel: w370 -> [w375 w377]
          tunnel: [w374 w376] -> w369
          frame "Idle", Default {
            n118 = call <vilib>:"Unset Busy.vi"("error in (no error)"=w375) -> ("error out"=w374:errorcluster)  [unwired: 10 in]
          }
          frame "Busy" {
            n119 = call <vilib>:"Set Busy.vi"("error in (no error)"=w377) -> ("error out"=w376:errorcluster)  [unwired: 9 in, 1 out]
          }
        }
        n120 = call <vilib>:"Add State(s) to Queue__JKI_lib_State_Machine.vi"("State(s) in (\"\")"=w373) -> ("States Out"=w372:string)  [unwired: 14 in]
      }
      frame "UI: Front Panel State" {
        # "Argument"
        # "Set Front Panel Open or Closed\n(Usage: \"UI: Front Panel State >> Open|Close\")"
        n121 = Unbundle By Name(w382) -> ("Core.Current VI Reference"=w381:refnum<vi>)
        n122 = case shown="\"Close\", \"Closed\"" w380 {
          tunnel: w384 -> [w392 w407 w418 w431 w444]
          tunnel: [w394 w408 w420 w433 w446] -> w383
          tunnel: w381 -> [w393 w405 w419 w432 w445]
          frame "Open", "Standard", Default {
            w387 = T4."Standard" ("State")
            n123 = property class="VI"(reference=w393, error in=w392) -> (reference out=w390:refnum<vi>, error out=w391:errorcluster, "FP.State"=w389:T4)
            n124 = Not Equal?(x=w389, y=w387) -> (x != y?=w388:bool)
            n125 = case shown="True" w388 {
              tunnel: [w398 w400] -> w394
              tunnel: w391 -> [w397 w400]
              tunnel: w390 -> [w396 _]
              tunnel: w387 -> [w395 _]
              frame True {
                n126 = invoke class="VI" method="FP.Open"(reference=w396, error in=w397, "Activate"=FALSE, "State"=w395) -> (error out=w398:errorcluster)  [unwired: 1 in, 4 out]
              }
              frame False {
              }
            }
          }
          frame "Close", "Closed" {
            n127 = property class="VI"(reference=w405, error in=w407) -> (reference out=w404:refnum<vi>, error out=w406:errorcluster, "FP.State"=w402:T4)
            n128 = Not Equal?(x=w402, y=T4."Closed" ("Front Panel Window:State")) -> (x != y?=w401:bool)
            n129 = case shown="True" w401 {
              tunnel: [w409 w412] -> w408
              tunnel: w406 -> [w409 w411]
              tunnel: w404 -> [_ w410]
              frame False {
              }
              frame True {
                n130 = invoke class="VI" method="FP.Close"(reference=w410, error in=w411) -> (error out=w412:errorcluster)  [unwired: 1 in, 2 out]
              }
            }
          }
          frame "Hidden", "Hide" {
            w413 = T4."Hidden" ("State")
            n131 = property class="VI"(reference=w419, error in=w418) -> (reference out=w416:refnum<vi>, error out=w417:errorcluster, "FP.State"=w415:T4)
            n132 = Not Equal?(x=w415, y=w413) -> (x != y?=w414:bool)
            n133 = case shown="True" w414 {
              tunnel: [w424 w425] -> w420
              tunnel: w417 -> [w423 w425]
              tunnel: w416 -> [w422 _]
              tunnel: w413 -> [w421 _]
              frame True {
                n134 = invoke class="VI" method="FP.Open"(reference=w422, error in=w423, "State"=w421) -> (error out=w424:errorcluster)  [unwired: 2 in, 4 out]
              }
              frame False {
              }
            }
          }
          frame "Minimize", "Minimized" {
            w426 = T4."Minimized" ("State")
            n135 = property class="VI"(reference=w432, error in=w431) -> (reference out=w429:refnum<vi>, error out=w430:errorcluster, "FP.State"=w428:T4)
            n136 = Not Equal?(x=w428, y=w426) -> (x != y?=w427:bool)
            n137 = case shown="True" w427 {
              tunnel: [w437 w438] -> w433
              tunnel: w430 -> [w436 w438]
              tunnel: w429 -> [w435 _]
              tunnel: w426 -> [w434 _]
              frame True {
                n138 = invoke class="VI" method="FP.Open"(reference=w435, error in=w436, "State"=w434) -> (error out=w437:errorcluster)  [unwired: 2 in, 4 out]
              }
              frame False {
              }
            }
          }
          frame "Maximize", "Maximized" {
            w439 = T4."Maximized" ("State")
            n139 = property class="VI"(reference=w445, error in=w444) -> (reference out=w442:refnum<vi>, error out=w443:errorcluster, "FP.State"=w441:T4)
            n140 = Not Equal?(x=w441, y=w439) -> (x != y?=w440:bool)
            n141 = case shown="True" w440 {
              tunnel: [w450 w451] -> w446
              tunnel: w443 -> [w449 w451]
              tunnel: w442 -> [w448 _]
              tunnel: w439 -> [w447 _]
              frame True {
                n142 = invoke class="VI" method="FP.Open"(reference=w448, error in=w449, "State"=w447) -> (error out=w450:errorcluster)  [unwired: 2 in, 4 out]
              }
              frame False {
              }
            }
          }
        }
        n143 = call <vilib>:"Add State(s) to Queue__JKI_lib_State_Machine.vi"("State(s) in (\"\")"=w386) -> ("States Out"=w385:string)  [unwired: 14 in]
      }
      frame "---------- Event Mode ----------" {
        # "Event Mode Separator"
        n144 = call <vilib>:"Add State(s) to Queue__JKI_lib_State_Machine.vi"("State(s) in (\"\")"=w457) -> ("States Out"=w456:string)  [unwired: 14 in]
      }
      frame "Event Mode: Data Init" {
        w468 = FALSE  # Stop Pressed?
        w466 = u32 0  # Iteration Count
        w471 = path ""  # Dump txt file path
        w467 = 0.0  # Start Time
        # "Initialize the data to be used in the event mode"
        n145 = invoke on="FITS File Generated?" class="Bool (strict)" method="Reinit To Default"(error in=w463) -> (error out=w462:errorcluster)  [unwired: 2 in, 2 out]
        n146 = invoke on="Iteration Count" class="DigNum (strict)" method="Reinit To Default"(error in=w462) -> (error out=w461:errorcluster)  [unwired: 2 in, 2 out]
        n147 = call "csvHeaderGen.vi"() -> ("Valid Data in Buffer"=w470:i32, "Data Buffer"=w469:string)  [unwired: 10 in]
        n148 = Bundle By Name(cluster=w465, "Stop Pressed?"=w468, "Start Time"=w467, "Iteration Count"=w466, "CSV File Data.Dump txt file path"=w471, "CSV File Data.Data Buffer"=w469, "CSV File Data.Valid Data in Buffer"=w470) -> (w464:T8)
        n149 = invoke on="Time elapsed" class="DigNum (strict)" method="Reinit To Default"(error in=w461) -> (error out=w458:errorcluster)  [unwired: 2 in, 2 out]
        n150 = invoke on="Event Mode" class="Bool (strict)" method="Reinit To Default"(error in=w458) -> (error out=w460:errorcluster)  [unwired: 2 in, 2 out]
        n151 = call <vilib>:"Add State(s) to Queue__JKI_lib_State_Machine.vi"("State(s) in (\"\")"=w474) -> ("States Out"=w473:string)  [unwired: 14 in]
      }
      frame "Event Mode: Data Get" {
        # "Template Separator\n(You can make a copy of, or modify, this frame)"
        n152 = Unbundle("Acquisition Period") -> ("Hours"=w481:u32, "Minutes"=w490:u32, "Seconds"=w488:u32)
        n153 = expression code="x*3600"(w481) -> (w482:u32)
        n154 = expression code="x*60"(w490) -> (w489:u32)
        n155 = property on="CZT 2 Threshold" class="DigNum (strict)"(error in=w483) -> (error out=w477:errorcluster, "Value"=w484:u16)  [unwired: 1 in, 1 out]
        n156 = Compound Arithmetic op=ADD(w482, w489, w488) -> (w487:u32)
        n157 = Bundle("User Name"="User Name", "Short Description"="Short Description", "Test Description"="Test Description", "Value"=w484) -> (w476:T13)  [unwired: 1 in]
        n158 = Bundle By Name(cluster=w480, "Acquisition Period"=w487, "User & Config Data"=w476) -> (w479:T8)
        n159 = call <vilib>:"Add State(s) to Queue__JKI_lib_State_Machine.vi"("State(s) in (\"\")"=w494) -> ("States Out"=w493:string)  [unwired: 14 in]
      }
      frame "Event Mode: Data Verif" {
        # "Checks if all the required data has been entered by the user! If all okay them moves to next state as per macro."
        # "Verify the data entered by the user if it is within its limits"
        n160 = Unbundle By Name(w508) -> ("User & Config Data.Description"=w500:string, "Acquisition Period"=w506:dbl, "User & Config Data.User Name"=w505:string, "User & Config Data.Short Description"=w504:string, "User & Config Data.Current Threshold Value"=w503:u16)
        n161 = call "chkEvntSet.vi"("Description"=w500, "Acquisition Period"=w506, "error in (no error)"=w509, "Current Threshold Value"=w503, "Short Description"=w504, "User Name"=w505) -> ("error out"=w498:errorcluster)  [unwired: 5 in]
        n162 = Select(t="", s=w498, f=w502) -> (s? t:f=w495:string)
        n163 = property on="Stop" class="Bool (strict)"(error in=w498, "DisabledEnum"=T6."Enabled" ("Disabled")) -> (error out=w497:errorcluster)  [unwired: 1 in, 1 out]
        n164 = call <vilib>:"Add State(s) to Queue__JKI_lib_State_Machine.vi"("State(s) in (\"\")"=w495) -> ("States Out"=w510:string)  [unwired: 14 in]
      }
      frame "Event Mode: Send Cmd" {
        # "Send the Event mode start command and start recieving the code"
        n165 = property on="Stop" class="Bool (strict)"(error in=w513) -> (error out=w512:errorcluster, "Value"=w511:bool)  [unwired: 1 in, 1 out]
        n166 = case shown="False" w511 {
          selector: w511 -> [_ w555]
          tunnel: w520 -> [w552 w560]
          tunnel: [w551 w560] -> w519
          tunnel: w512 -> [w525 w557]
          tunnel: [w548 w554] -> w518
          tunnel: [w547 "Event Mode: Close CSV"] -> w517
          tunnel: [w537 _] -> w516
          tunnel: w515 -> [w538 w553]
          tunnel: [w523 w556] -> w514
          frame False {
            w528 = "¡ÿU"  # Event mode ON with Emulator
            w529 = " ÿU"  # Event mode ON w/o Emulator
            # "Generate the dump file name and create storage directory"
            # "If there is no error log current timer value"
            n167 = Unbundle(w538) -> ("Acquisition Period"=w530:dbl, "CSV File Data"=w543:T11, "User & Config Data"=w541:T10)  [unwired: 5 out]
            n168 = Unbundle(w541) -> ("User Name"=w533:string, "Short Description"=w532:string, "Current Threshold Value"=w531:u16)  [unwired: 1 out]
            n169 = Get Date/Time In Seconds() -> (seconds since 1Jan1904=w534:timestamp)
            n170 = call "csvNameGenerate.vi"("User Name"=w533, "time stamp"=w534, "Short Description"=w532, "Threshold Value"=w531, "Acquisition Period"=w530, "error in"=w525) -> ("Dump file path"=w535:path, "Byte Stream File out"=w537:refnum<file>, "File Name"=w536:string, "error out"=w524:errorcluster)  [unwired: 6 in]
            n171 = Select(t=w528, s="Emulate?", f=w529) -> (s? t:f=w527:string)
            n172 = Bundle(cluster=w543, "Dump txt file path"=w535, "Fits File name"=w536, "Test Start time"=w534) -> (w542:T11)  [unwired: 3 in]
            n173 = VISA Write(VISA resource name=w552, write buffer=w527, error in (no error)=w524) -> (VISA resource name out=w551:refnum<visa-resource-name>, return count=w540:u32, error out=w523:errorcluster)
            n174 = Greater Than 0?(x=w540) -> (x > 0?=→"Event Mode":bool)
            n175 = call <vilib>:"High Resolution Relative Seconds.vi"() -> ("relative seconds"=w546:dbl)
            n176 = Select(t=0.0, s=w523, f=w546) -> (s? t:f=w545:dbl)
            n177 = Select(t="", s=w523, f="Event Mode: Rec Data") -> (s? t:f=w547:string)
            n178 = Bundle(cluster=w538, "Start Time"=w545, "CSV File Data"=w542) -> (w548:T8)  [unwired: 6 in]
          }
          frame True {
            n179 = Bundle By Name(cluster=w553, "Stop Pressed?"=w555) -> (w554:T8)
            n180 = property on="Stop" class="Bool (strict)"(error in=w557, "Value"=FALSE ("Stop")) -> (error out=w556:errorcluster)  [unwired: 1 in, 1 out]
          }
        }
        n181 = call <vilib>:"Add State(s) to Queue__JKI_lib_State_Machine.vi"("State(s) in Front (\"\")"=w517, "State(s) in (\"\")"=w522) -> ("States Out"=w521:string)  [unwired: 13 in]
      }
      frame "Event Mode: Rec Data" {
        # "Check if the stop button is pressed, each loop"
        # "Record the event mode data into a csv file"
        n182 = case shown="False" "Stop" {
          selector: "Stop" -> [_ w629]
          tunnel: [w605 "Event Mode: Close CSV"] -> w570
          tunnel: w569 -> [w604 w634]
          tunnel: w568 -> [w603 w632]
          tunnel: [w602 w634] -> w567
          tunnel: [w573 w630] -> w566
          tunnel: w565 -> [w600 w635]
          tunnel: [w599 w635] -> w564
          tunnel: [w585 w627] -> w563
          tunnel: w562 -> [w597 w628]
          frame False {
            # "#Modify the formatter format here"
            # "Write formatted data to the dump txt file"
            # "Format input data as per csv"
            # "Elapsed time generation & comparison logic"
            n183 = Unbundle(w597) -> ("Start Time"=w610:dbl, "Acquisition Period"=w608:dbl, "Iteration Count"=w580:u32, "CSV File Data"=w594:T11)  [unwired: 4 out]
            "Iteration Count" <- w580
            n184 = call <vilib>:"High Resolution Relative Seconds.vi"() -> ("relative seconds"=w609:dbl)
            n185 = VISA Read(VISA resource name=w604, byte count=u32 50, error in (no error)=w603) -> (VISA resource name out=w602:refnum<visa-resource-name>, read buffer=w582:string, error out=w598:errorcluster)  [unwired: 1 out]
            "read buffer" <- w582
            n186 = Subtract(x=w609, y=w610) -> (x-y=w601:dbl)
            "Time elapsed" <- w601
            n187 = Less?(x=w601, y=w608) -> (x < y?=w578:bool)
            n188 = call "csvFormatter.vi"("Iteration"=w580, "error in (no error)"=w598, "Sensor Data In"=w582) -> ("error out"=w596:errorcluster, "CSV formatted String"=w595:string)  [unwired: 7 in]
            n189 = Unbundle(w594) -> ("Dump txt file path"=w590:path, "Data Buffer"=w592:string, "Valid Data in Buffer"=w593:i32, "CSV file path"=w586:path, "Fits File name"=w584:string, "Test Start time"=w583:timestamp)
            n190 = disable-structure shown="Enabled" {
              disable-tunnel: w600 -> [w619 w623]
              disable-tunnel: [w618 w624] -> w599
              disable-tunnel: w596 -> [w617 w626]
              disable-tunnel: w595 -> [w616 w622]
              disable-tunnel: w593 -> [w615 w621]
              disable-tunnel: w592 -> [w614 w620]
              disable-tunnel: [w613 w620] -> w589
              disable-tunnel: [w612 w621] -> w588
              disable-tunnel: [w611 w625] -> w574
              frame Enabled {
                n191 = call "csvBitWrite.vi"("data buffer"=w614, "valid data in buffer"=w615, "error in (no error)"=w617, "CSV Formatted String"=w616, "Byte Stream File in"=w619) -> ("error out"=w611:errorcluster, "Valid Data Buf OUT"=w612:i32, "Data buffer OUT"=w613:string, "Byte Stream File out"=w618:refnum<file>)  [unwired: 3 in]
              }
              frame Disabled {
                n192 = Write to Text File(file (use dialog)=w623, text=w622, error in=w626) -> (refnum out=w624:refnum<file>, error out=w625:errorcluster)  [unwired: 1 in, 1 out]
              }
            }
            n193 = Increment(x=w580) -> (x+1=w591:u32)
            n194 = Bundle("Dump txt file path"=w590, "Data buffer OUT"=w589, "Valid Data Buf OUT"=w588, "CSV file path"=w586, "Fits File name"=w584, "Test Start time"=w583) -> (w587:T14)  [unwired: 1 in]
            n195 = Bundle(cluster=w597, "Iteration Count"=w591, "CSV File Data"=w587) -> (w585:T8)  [unwired: 6 in]
            n196 = call <vilib>:"Clear Errors.vi"("error in (no error)"=w574, "specific error code to clear (0: all)"=-1073807339) -> ("error out"=w573:errorcluster)  [unwired: 4 in, 1 out]
            n197 = Less?(x=w580, y="Iteration Limit") -> (x < y?=w579:bool)
            n198 = And(x=w578, y=w579) -> (x .and. y?=w577:bool)
            n199 = Select(t="Event Mode: Rec Data", s=w577, f="Event Mode: Close CSV") -> (s? t:f=w605:string)
          }
          frame True {
            # "Latched button resetted"
            # "Stop button Pressed; End data acquisition"
            n200 = Bundle By Name(cluster=w628, "Stop Pressed?"=w629) -> (w627:T8)
            n201 = property on="Stop" class="Bool (strict)"(error in=w632, "Value"=FALSE ("Stop")) -> (error out=w630:errorcluster)  [unwired: 1 in, 1 out]
          }
        }
        n202 = call <vilib>:"Add State(s) to Queue__JKI_lib_State_Machine.vi"("State(s) in Front (\"\")"=w570, "State(s) in (\"\")"=w572) -> ("States Out"=w571:string)  [unwired: 13 in]
      }
      frame "Event Mode: Close CSV" {
        # "#Remove the En/Dis block before testing"
        # "Change dump file extension to csv"
        # "Close file ref"
        # "Write last line of data"
        # "Close the reference to the CSV file and change the extension from .txt to .csv"
        n203 = Unbundle(w651) -> ("CSV File Data"=w647:T11)  [unwired: 7 out]
        n204 = disable-structure shown="Enabled" {
          disable-tunnel: w644 -> [w673 w676]
          disable-tunnel: w643 -> [w672 w675]
          disable-tunnel: [w671 w676] -> w642
          disable-tunnel: [w670 w675] -> w637
          frame Disabled {
            w674 = " \u0000U"  # Event mode OFF
            n205 = VISA Write(VISA resource name=w673, write buffer=w674, error in (no error)=w672) -> (VISA resource name out=w671:refnum<visa-resource-name>, error out=w670:errorcluster)  [unwired: 1 out]
          }
          frame Enabled {
          }
        }
        n206 = Unbundle(w647) -> ("Data Buffer"=w649:string, "Valid Data in Buffer"=w648:i32)  [unwired: 4 out]
        n207 = String Subset(string=w649, length (rest)=w648) -> (substring=w660:string)  [unwired: 1 in]
        n208 = disable-structure shown="Enabled" {
          disable-tunnel: w660 -> [w667 _]
          disable-tunnel: w659 -> [w666 w669]
          disable-tunnel: [w665 w668] -> w658
          disable-tunnel: [w664 w669] -> w657
          disable-tunnel: w643 -> [w663 w668]
          frame Enabled {
            n209 = Write to Text File(file (use dialog)=w666, text=w667, error in=w663) -> (refnum out=w664:refnum<file>, error out=w665:errorcluster)  [unwired: 1 in, 1 out]
          }
          frame Disabled {
          }
        }
        n210 = Close File(refnum=w657, error in=w658) -> (path=w639:path, error out=w656:errorcluster)
        n211 = call "changeEXT.vi"("Path"=w639, "error in (no error)"=w656, "New Extension"="csv") -> ("error out"=w641:errorcluster, "Success?"=w638:bool, "Out CSV Path"=w646:path)  [unwired: 6 in]
        n212 = Bundle(cluster=w647, "CSV file path"=w646) -> (w645:T11)  [unwired: 5 in]
        n213 = invoke on="Event Mode" class="Bool (strict)" method="Reinit To Default"(error in=w637) -> (error out=w636:errorcluster)  [unwired: 2 in, 2 out]
        n214 = Bundle(cluster=w651, "CSV File Data"=w645) -> (w650:T8)  [unwired: 7 in]
        n215 = Select(t="Event Mode: Make FITS", s=w638, f="") -> (s? t:f=w654:string)
        n216 = Merge Errors(w636, w641) -> (w640:errorcluster)
        n217 = call <vilib>:"Add State(s) to Queue__JKI_lib_State_Machine.vi"("State(s) in Front (\"\")"=w654, "State(s) in (\"\")"=w662) -> ("States Out"=w661:string)  [unwired: 13 in]
      }
      frame "Event Mode: Make FITS" {
        # "FITS Metadata Requirement:\n>File name // Str- Done\n>Date Time //Str -done\n>User Name //Str - Done\n>Comments //Str - done\n>Original File Path //Str-done\n>Threshold Value //Int-done\n>Pixel data //Str-done\n>Acquisition Period //Str-done"
        # "Calls a python function to convert the .csv file to a .fits file"
        n218 = Unbundle By Name(w696) -> ("CSV File Data.CSV file path"=w688:path, "CSV File Data.Fits File name"=w689:string, "User & Config Data.User Name"=w693:string, "User & Config Data.Short Description"=w692:string, "User & Config Data.Description"=w684:string, "CSV File Data.Test Start time"=w685:timestamp, "Acquisition Period"=w691:dbl, "User & Config Data.Current Threshold Value"=w686:u16, "Pixel Status.Disabled Pixels"=w687:u8[])
        n219 = property on="Stop" class="Bool (strict)"(error in=w681, "DisabledEnum"=T6."Disabled and Grayed Out" ("Disabled")) -> (error out=w680:errorcluster)  [unwired: 1 in, 1 out]
        n220 = Bundle("Fits File name"=w689, "User Name"=w693, "Short Description"=w692, "Description"=w684, "Test Start time"=w685, "Acquisition Period"=w691, "Current Threshold Value"=w686, "Disabled Pixels"=w687) -> (w683:T15)  [unwired: 1 in]
        n221 = call "convertFITS.vi"("error in (no error)"=w680, "Header data cluster"=w683, "Input CSV File path"=w688) -> ("error out"=w678:errorcluster, "Success?"=→"FITS File Generated?":bool)  [unwired: 6 in, 1 out]
        n222 = property on="Open CSV" class="Bool"(error in=w678, "DisabledEnum"=T6."Enabled" ("Disabled")) -> (error out=w677:errorcluster)  [unwired: 1 in, 1 out]
        n223 = call <vilib>:"Add State(s) to Queue__JKI_lib_State_Machine.vi"("State(s) in Front (\"\")"="Event Mode: Update Graphs", "State(s) in (\"\")"=w699) -> ("States Out"=w698:string)  [unwired: 13 in]
      }
      frame "Event Mode: Update Graphs" {
        w700 = u8[] [0, 1, 2, 3, 4, 5, 6, 7, 8, 9, 10, 11, 12, 13, 14, 15, 0, 1, 2, 3, 4, 5, 6, 7, 8, 9, 10, 11, 12, 13, 14, 15, 0, 1, 2, 3, 4, 5, 6, 7, 8, 9, 10, 11, 12, 13, 14, 15, 0, 1, 2, 3, 4, 5, 6, 7, 8, 9, 10, 11, 12, 13, 14, 15, 0, 1, 2, 3, 4, 5, 6, 7, 8, 9, 10, 11, 12, 13, 14, 15, 0, 1, 2, 3, 4, 5, 6, 7, 8, 9, 10, 11, 12, 13, 14, 15, 0, 1, 2, 3, 4, 5, 6, 7, 8, 9, 10, 11, 12, 13, 14, 15, 0, 1, 2, 3, 4, 5, 6, 7, 8, 9, 10, 11, 12, 13, 14, 15, 0, 1, 2, 3, 4, 5, 6, 7, 8, 9, 10, 11, 12, 13, 14, 15, 0, 1, 2, 3, 4, 5, 6, 7, 8, 9, 10, 11, 12, 13, 14, 15, 0, 1, 2, 3, 4, 5, 6, 7, 8, 9, 10, 11, 12, 13, 14, 15, 0, 1, 2, 3, 4, 5, 6, 7, 8, 9, 10, 11, 12, 13, 14, 15, 0, 1, 2, 3, 4, 5, 6, 7, 8, 9, 10, 11, 12, 13, 14, 15, 0, 1, 2, 3, 4, 5, 6, 7, 8, 9, 10, 11, 12, 13, 14, 15, 0, 1, 2, 3, 4, 5, 6, 7, 8, 9, 10, 11, 12, 13, 14, 15, 0, 1, 2, 3, 4, 5, 6, 7, 8, 9, 10, 11, 12, 13, 14] ("Array")
        # "Reads the event data and updates the graphs"
        n224 = Unbundle By Name(w711) -> ("CSV File Data.CSV file path"=w710:path)
        n225 = call-poly <vilib>:"Read Delimited Spreadsheet.vi"("file path (dialog if empty)"=w710, "error in (no error)"=w707, "delimiter (\\t)"=",") -> ("all rows"=w719:string[][], "error out"=w708:errorcluster)  [unwired: 7 in, 4 out]
        "all rows" <- w719
        n226 = Array Subset(array=w719, index (row)=1 ("index")) -> (w717:string[][])  [unwired: 3 in]
        n227 = Index Array(array=w717, index (col)=4 ("disabled index (col)")) -> (element=w715:string[])  [unwired: 1 in]
        n228 = Hexadecimal String To Number(string=w715) -> (number=w713:u32[])  [unwired: 2 in, 1 out]
        n229 = call <vilib>:"Histogram.vi"("intervals"=255, "X"=w713) -> ("Histogram Graph"=→"Event Count Histogram":T1)  [unwired: 5 in, 4 out]
        n230 = call "mapEventCounts.vi"("Count"=w713) -> ("Counts (map)"=w701:map{u32, u32}, "Count Grid"=w705:u32[][])  [unwired: 3 in]
        n231 = call "mapTo2DArr.vi"("Map"=w701) -> ("2D Array"=w702:i32[][])
        n232 = Transpose 2D Array(2D array=w705) -> (transposed array=→"Intensity Graph":u32[][])
        n233 = call "sort2DArrayAscDesc.vi"("2D Array"=w702) -> ("sorted 2D array"=→"Noisy Pixel List":i32[][])  [unwired: 5 in]
        n234 = call-poly <vilib>:"Plot Helper.vi"("z matrix"=w705, "error in (no error)"=w708, "y vector"=w700, "x vector"=w700) -> ("error out"=w706:errorcluster, "3D Plot lvclass Array out"=→"Detector Surface":refnum<class "3D Plot Datatype.lvclass">[])  [unwired: 2 in, 4 out]
        n235 = call <vilib>:"Add State(s) to Queue__JKI_lib_State_Machine.vi"("State(s) in Front (\"\")"="UART Comm: Close", "State(s) in (\"\")"=w725) -> ("States Out"=w724:string)  [unwired: 13 in]
      }
      frame "---------- Pixel Status ----------" {
        # "Pixel Status Separator"
        n236 = call <vilib>:"Add State(s) to Queue__JKI_lib_State_Machine.vi"("State(s) in (\"\")"=w731) -> ("States Out"=w730:string)  [unwired: 14 in]
      }
      frame "Pixel Status: Pix Send On" {
        # "Sends the command to the FPGA to toggle the status of the Pixel"
        n237 = Number To Hexadecimal String(1:i16 2 ("width (-)"), 2:"Choose Pixel To Toggle") -> (0:w741:string)
        n238 = call "hexStrConv.vi"("Input ASCII Hex String"=w741, "error in (no error)"=w733) -> ("Output Non Printable HEX String"=w740:string, "error out"=w735:errorcluster)  [unwired: 1 out]
        n239 = Concatenate Strings("Ð", w740, "U") -> (w736:string)
        n240 = VISA Write(VISA resource name=w743, write buffer=w736, error in (no error)=w735) -> (VISA resource name out=w737:refnum<visa-resource-name>, error out=w734:errorcluster)  [unwired: 1 out]
        n241 = call <vilib>:"Add State(s) to Queue__JKI_lib_State_Machine.vi"("State(s) in (\"\")"=w747) -> ("States Out"=w746:string)  [unwired: 14 in]
      }
      frame "Pixel Status: Pix Send Off" {
        # "Sends the command to the FPGA to toggle the status of the Pixel"
        n242 = property on="Choose Pixel To Toggle" class="DigNum (strict)"(error in=w752) -> (error out=w750:errorcluster, "Value"=w751:u8)  [unwired: 1 in, 1 out]
        n243 = Number To Hexadecimal String(1:i16 2 ("width (-)"), 2:w751) -> (0:w759:string)
        n244 = call "hexStrConv.vi"("Input ASCII Hex String"=w759, "error in (no error)"=w750) -> ("Output Non Printable HEX String"=w758:string, "error out"=w753:errorcluster)  [unwired: 1 out]
        n245 = Concatenate Strings("Ñ", w758, "U") -> (w754:string)
        n246 = VISA Write(VISA resource name=w760, write buffer=w754, error in (no error)=w753) -> (VISA resource name out=w755:refnum<visa-resource-name>, error out=w748:errorcluster)  [unwired: 1 out]
        n247 = case shown="No Error" w748 {
          frame No Error {
          }
          frame Error {
          }
        }
        n248 = call <vilib>:"Add State(s) to Queue__JKI_lib_State_Machine.vi"("State(s) in (\"\")"=w764) -> ("States Out"=w763:string)  [unwired: 14 in]
      }
      frame "Pixel Status: Pix Rec" {
        w776 = "D%1x%2x" ("format string")
        # "Recieves the data from the FPGA whether the operation has been sucessfully performed or not"
        n249 = VISA Read(VISA resource name=w789, byte count=u32 16, error in (no error)=w787) -> (VISA resource name out=w788:refnum<visa-resource-name>, read buffer=w783:string, error out=w773:errorcluster)  [unwired: 1 out]
        n250 = call <vilib>:"Trim Whitespace.vi"("string"=w783) -> ("trimmed string"=w779:string)  [unwired: 1 in]
        n251 = Search/Split String(string=w779, search string/char (-)="\t") -> (substring before match=w778:string, match + rest of string=w782:string)  [unwired: 1 in, 1 out]
        n252 = String Subset(string=w782, offset (0)=1) -> (substring=w777:string)  [unwired: 1 in]
        n253 = call "pixStatusConvert.vi"("format string"=w776, "error in"=w773, "Hex Input String"=w777) -> ("error out"=w772:errorcluster, "Pix No."=w766:u16, "En/Dis?"=w774:bool)  [unwired: 6 in]
        n254 = call "pixStatusConvert.vi"("format string"=w776, "error in"=w773, "Hex Input String"=w778) -> ("error out"=w771:errorcluster, "Pix No."=w767:u16, "En/Dis?"=w775:bool)  [unwired: 6 in]
        n255 = Merge Errors(w771, w772) -> (w770:errorcluster)
        n256 = Select(t=w775, s="Detector Chooser", f=w774) -> (s? t:f=w769:bool)
        n257 = Select(t=w767, s="Detector Chooser", f=w766) -> (s? t:f=w768:u16)
        n258 = Bundle By Name(cluster=w785, "Pixel Status.Pixel En/Dis?"=w769, "Pixel Status.Pixel Number"=w768) -> (w786:T8)
        n259 = call <vilib>:"Add State(s) to Queue__JKI_lib_State_Machine.vi"("State(s) in (\"\")"=w792) -> ("States Out"=w791:string)  [unwired: 14 in]
      }
      frame "Pixel Status: Update Pix Matrix" {
        # "Updates the Pixel matrix UI"
        n260 = Unbundle By Name(w799) -> ("Pixel Status.Pixel Array"=w802:bool[][], "Pixel Status.Pixel Number"=w796:u16, "Pixel Status.Pixel En/Dis?"=w797:bool, "Pixel Status"=w795:T9)
        n261 = call "noToCoord.vi"("Pixel number"=w796) -> ("i"=w801:u8, "j"=w800:u8)  [unwired: 6 in]
        n262 = Replace Array Subset(array=w802, new element=w797, index (row)=w801, index (col)=w800) -> (w798:bool[][])
        "Pixel Matrix Status" <- w798
        n263 = call "addRemDisList.vi"("Pixel Status"=w795) -> ("Disabled Pixels"=w793:u8[])  [unwired: 10 in]
        n264 = Bundle By Name(cluster=w799, "Pixel Status.Pixel Array"=w798, "Pixel Status.Disabled Pixels"=w793) -> (w794:T8)
        n265 = call <vilib>:"Add State(s) to Queue__JKI_lib_State_Machine.vi"("State(s) in (\"\")"=w807) -> ("States Out"=w806:string)  [unwired: 14 in]
      }
      frame "---------- All Pixel Status ----------" {
        # "All Pixel Status Separator"
        n266 = call <vilib>:"Add State(s) to Queue__JKI_lib_State_Machine.vi"("State(s) in (\"\")"=w813) -> ("States Out"=w812:string)  [unwired: 14 in]
      }
      frame "All Pixel Status: Pix Send All" {
        n267 = VISA Write(VISA resource name=w818, write buffer="ß\u0000", error in (no error)=w816) -> (VISA resource name out=w817:refnum<visa-resource-name>, error out=w815:errorcluster)  [unwired: 1 out]
        n268 = call <vilib>:"Add State(s) to Queue__JKI_lib_State_Machine.vi"("State(s) in (\"\")"=w822) -> ("States Out"=w821:string)  [unwired: 14 in]
      }
      frame "All Pixel Status: Pix Rec All" {
        n269 = disable-structure shown="Enabled" {
          disable-tunnel: [w844 w853] -> w834
          disable-tunnel: w833 -> [w843 w853]
          disable-tunnel: w832 -> [w842 w848]
          disable-tunnel: [w838 w846] -> w830
          disable-tunnel: [w841 w847] -> w829
          frame Disabled {
            n270 = VISA Read(VISA resource name=w843, byte count=u32 16, error in (no error)=w842) -> (VISA resource name out=w844:refnum<visa-resource-name>, read buffer=w839:string, error out=w841:errorcluster)  [unwired: 1 out]
            n271 = call <vilib>:"Trim Whitespace.vi"("string"=w839) -> ("trimmed string"=w838:string)  [unwired: 1 in]
          }
          frame Enabled {
            n272 = Number To Hexadecimal String(1:2, 2:128) -> (0:w850:string)
            n273 = call "hexStrConv.vi"("Input ASCII Hex String"=w850, "error in (no error)"=w848) -> ("Output Non Printable HEX String"=w851:string, "error out"=w847:errorcluster)  [unwired: 1 out]
            n274 = Concatenate Strings("Ð", w851) -> (w846:string)
          }
        }
        n275 = call "pixStatusConvert.vi"("format string"="D%1x%2x", "error in"=w829, "Hex Input String"=w830) -> ("error out"=w828:errorcluster, "Pix No."=w826:u16, "En/Dis?"=w827:bool)  [unwired: 6 in]
        n276 = Bundle By Name(cluster=w825, "Pixel Status.Pixel En/Dis?"=w827, "Pixel Status.Pixel Number"=w826) -> (w824:T8)
        n277 = call <vilib>:"Add State(s) to Queue__JKI_lib_State_Machine.vi"("State(s) in Front (\"\")"="All Pixel Status: Update Matrix", "State(s) in (\"\")"=w837) -> ("States Out"=w836:string)  [unwired: 13 in]
      }
      frame "All Pixel Status: Update Matrix" {
        n278 = Unbundle By Name(w864) -> ("Pixel Status.Pixel Array"=w865:bool[][], "Pixel Status.Pixel Number"=w854:u16, "Pixel Status.Pixel En/Dis?"=w867:bool, "Pixel Status"=w868:T9)
        n279 = call "noToCoord.vi"("Pixel number"=w854) -> ("i"=w866:u8, "j"=w870:u8)  [unwired: 6 in]
        n280 = Replace Array Subset(array=w865, new element=w867, index (row)=w866, index (col)=w870) -> (w860:bool[][])
        n281 = call "addRemDisList.vi"("Pixel Status"=w868) -> ("Disabled Pixels"=w869:u8[])  [unwired: 10 in]
        n282 = Bundle By Name(cluster=w864, "Pixel Status.Pixel Array"=w860, "Pixel Status.Disabled Pixels"=w869) -> (w863:T8)
        n283 = property on="Pixel Matrix Status" class="Arr (strict)"(error in=w861, "Value"=w860) -> (error out=w862:errorcluster)  [unwired: 1 in, 1 out]
        n284 = Equal?(x=w854, y=255) -> (x = y?=w858:bool)
        n285 = Select(t="UART Comm: Close", s=w858, f="All Pixel Status: Pix Rec All") -> (s? t:f=w857:string)
        n286 = call <vilib>:"Add State(s) to Queue__JKI_lib_State_Machine.vi"("State(s) in Front (\"\")"=w857, "State(s) in (\"\")"=w874) -> ("States Out"=w873:string)  [unwired: 13 in]
      }
      frame "---------- Threshold ----------" {
        # "Threshold States Separator"
        n287 = call <vilib>:"Add State(s) to Queue__JKI_lib_State_Machine.vi"("State(s) in (\"\")"=w880) -> ("States Out"=w879:string)  [unwired: 14 in]
      }
      frame "Threshold: Set Thresh" {
        # "Template Separator\n(You can make a copy of, or modify, this frame)"
        n288 = call "threshConvert.vi"("error in"=w882, "Select Threshold Value"="Select Threshold Value") -> ("error out"=w887:errorcluster, "Threshold Frame"=w885:string)  [unwired: 8 in]
        n289 = Concatenate Strings(w885, "U" ("string")) -> (w883:string)
        n290 = VISA Write(VISA resource name=w881, write buffer=w883, error in (no error)=w887) -> (VISA resource name out=w888:refnum<visa-resource-name>, error out=w886:errorcluster)  [unwired: 1 out]
        n291 = call <vilib>:"Add State(s) to Queue__JKI_lib_State_Machine.vi"("State(s) in (\"\")"=w893) -> ("States Out"=w892:string)  [unwired: 14 in]
      }
      frame "Threshold: Get Thresh" {
        w899 = "E%x" ("format string")
        # "Template Separator\n(You can make a copy of, or modify, this frame)"
        n292 = VISA Read(VISA resource name=w910, byte count=u32 16, error in (no error)=w908) -> (VISA resource name out=w909:refnum<visa-resource-name>, read buffer=w896:string, error out=w903:errorcluster)  [unwired: 1 out]
        n293 = call "dataSplitter.vi"("Input"=w896) -> ("After \\t"=w894:string, "Before \\t"=w895:string)  [unwired: 2 in]
        n294 = call "getThreshConv.vi"("format string"=w899, "error in (no error)"=w903, "Input HEX Threshold"=w894) -> ("error out"=w901:errorcluster, "Output Threshold Value"=→"CZT 2 Threshold":u16)  [unwired: 6 in, 1 out]
        n295 = call "getThreshConv.vi"("format string"=w899, "error in (no error)"=w903, "Input HEX Threshold"=w895) -> ("error out"=w902:errorcluster, "Output Threshold Value"=→"CZT 1 Threshold":u16)  [unwired: 6 in, 1 out]
        n296 = Merge Errors(w902, w901) -> (w900:errorcluster)
        n297 = Select(t="", s=w900, f=w904) -> (s? t:f=w905:string)
        n298 = call <vilib>:"Add State(s) to Queue__JKI_lib_State_Machine.vi"("State(s) in Front (\"\")"=w905, "State(s) in (\"\")"=w914) -> ("States Out"=w913:string)  [unwired: 13 in]
      }
      frame "---------- Emulator ----------" {
        # "Threshold States Separator"
        n299 = call <vilib>:"Add State(s) to Queue__JKI_lib_State_Machine.vi"("State(s) in (\"\")"=w920) -> ("States Out"=w919:string)  [unwired: 14 in]
      }
      frame "Emulator: Set Mode" {
        # "Template Separator\n(You can make a copy of, or modify, this frame)"
        n300 = property on="Emulate?" class="Bool (strict)"(error in=w926) -> (error out=w925:errorcluster, "Value"=w923:bool)  [unwired: 1 in, 1 out]
        n301 = Select(t="¡ÿU" ("string"), s=w923, f=" ÿU" ("string")) -> (s? t:f=w921:string)
        n302 = VISA Write(VISA resource name=w927, write buffer=w921, error in (no error)=w925) -> (VISA resource name out=w929:refnum<visa-resource-name>, error out=w928:errorcluster)  [unwired: 1 out]
        n303 = call <vilib>:"Add State(s) to Queue__JKI_lib_State_Machine.vi"("State(s) in (\"\")"=w933) -> ("States Out"=w932:string)  [unwired: 14 in]
      }
      frame "Emulator: Get Mode" {
        # "Check if the Emulator mode has been set and update LEDS accordingly"
        n304 = property on="Emulate?" class="Bool (strict)" props=["Value"](error in=w942) -> (error out=w941:errorcluster)  [unwired: 1 in, 2 out]
        n305 = disable-structure shown="Enabled" {
          disable-tunnel: w948 -> [w958 w960]
          disable-tunnel: [w957 w960] -> w947
          disable-tunnel: [w953 "1\t1"] -> w936
          disable-tunnel: [w956 w961] -> w943
          disable-tunnel: w941 -> [w955 w961]
          frame Enabled {
            n306 = VISA Read(VISA resource name=w958, byte count=u32 16, error in (no error)=w955) -> (VISA resource name out=w957:refnum<visa-resource-name>, read buffer=w953:string, error out=w956:errorcluster)  [unwired: 1 out]
          }
          frame Disabled {
          }
        }
        n307 = call "dataSplitter.vi"("Input"=w936) -> ("After \\t"=w934:string, "Before \\t"=w935:string)  [unwired: 2 in]
        n308 = Decimal String To Number(string=w934) -> (number=w937:i32)  [unwired: 2 in, 1 out]
        n309 = Decimal String To Number(string=w935) -> (number=w938:i32)  [unwired: 2 in, 1 out]
        n310 = Not Equal To 0?(x=w938) -> (x != 0?=→"Emulator 1":bool)
        n311 = Not Equal To 0?(x=w937) -> (x != 0?=→"Emulator 2":bool)
        n312 = Select(t="", s=w943, f=w944) -> (s? t:f=w945:string)
        n313 = call <vilib>:"Add State(s) to Queue__JKI_lib_State_Machine.vi"("State(s) in Front (\"\")"=w945, "State(s) in (\"\")"=w952) -> ("States Out"=w951:string)  [unwired: 13 in]
      }
      frame "---------- Serial Number ----------" {
        # "Serial Number States Separator"
        n314 = call <vilib>:"Add State(s) to Queue__JKI_lib_State_Machine.vi"("State(s) in (\"\")"=w967) -> ("States Out"=w966:string)  [unwired: 14 in]
      }
      frame "Serial Number: Send Command" {
        # "Template Separator\n(You can make a copy of, or modify, this frame)"
        n315 = call "hexStrConv.vi"("Input ASCII Hex String"="B000" ("format string"), "error in (no error)"=w970) -> ("Output Non Printable HEX String"=w968:string, "error out"=w969:errorcluster)  [unwired: 1 out]
        n316 = Concatenate Strings(w968, "U" ("string")) -> (w973:string)
        n317 = VISA Write(VISA resource name=w972, write buffer=w973, error in (no error)=w969) -> (VISA resource name out=w976:refnum<visa-resource-name>, error out=w975:errorcluster)  [unwired: 1 out]
        n318 = call <vilib>:"Add State(s) to Queue__JKI_lib_State_Machine.vi"("State(s) in (\"\")"=w980) -> ("States Out"=w979:string)  [unwired: 14 in]
      }
      frame "Serial Number: Get Number" {
        w981 = u32 0 ("default (0 U32)")
        w990 = T16 2 items=["both", "start of string", "end of string"] ("location (both)")
        # "Template Separator\n(You can make a copy of, or modify, this frame)"
        n319 = VISA Read(VISA resource name=w1001, byte count=u32 16, error in (no error)=w999) -> (VISA resource name out=w1000:refnum<visa-resource-name>, read buffer=w991:string, error out=w998:errorcluster)  [unwired: 1 out]
        n320 = call <vilib>:"Trim Whitespace.vi"("string"=w991, "location (both)"=w990) -> ("trimmed string"=w989:string)
        n321 = Search/Split String(string=w989, search string/char (-)="\t") -> (substring before match=w987:string, match + rest of string=w986:string)  [unwired: 1 in, 1 out]
        n322 = String Subset(string=w986, offset (0)=2) -> (substring=w984:string)  [unwired: 1 in]
        n323 = String Subset(string=w987, offset (0)=1) -> (substring=w993:string)  [unwired: 1 in]
        n324 = Hexadecimal String To Number(string=w984, default (0uL)=w981) -> (number=→"Serial Number 2":u32)  [unwired: 1 in, 1 out]
        n325 = Hexadecimal String To Number(string=w993, default (0uL)=w981) -> (number=→"Serial Number":u32)  [unwired: 1 in, 1 out]
        n326 = Select(t="", s=w998, f=w995) -> (s? t:f=w996:string)
        n327 = call <vilib>:"Add State(s) to Queue__JKI_lib_State_Machine.vi"("State(s) in Front (\"\")"=w996, "State(s) in (\"\")"=w1005) -> ("States Out"=w1004:string)  [unwired: 13 in]
      }
      frame "---------- Clock ----------" {
        # "Serial Number States Separator"
        n328 = call <vilib>:"Add State(s) to Queue__JKI_lib_State_Machine.vi"("State(s) in (\"\")"=w1011) -> ("States Out"=w1010:string)  [unwired: 14 in]
      }
      frame "Clock: Set Clock" {
        # "Template Separator\n(You can make a copy of, or modify, this frame)"
        n329 = Number To Hexadecimal String(1:i16 2 ("width (-)"), 2:"Set CZT Clock") -> (0:w1013:string)
        n330 = call "hexStrConv.vi"("Input ASCII Hex String"=w1013, "error in (no error)"=w1018) -> ("Output Non Printable HEX String"=w1016:string, "error out"=w1017:errorcluster)  [unwired: 1 out]
        n331 = Concatenate Strings("À", w1016, "U" ("string")) -> (w1020:string)
        n332 = VISA Write(VISA resource name=w1019, write buffer=w1020, error in (no error)=w1017) -> (VISA resource name out=w1023:refnum<visa-resource-name>, error out=w1022:errorcluster)  [unwired: 1 out]
        n333 = call <vilib>:"Add State(s) to Queue__JKI_lib_State_Machine.vi"("State(s) in (\"\")"=w1027) -> ("States Out"=w1026:string)  [unwired: 14 in]
      }
      frame "Clock: Get Clock" {
        w1042 = T16 2 items=["both", "start of string", "end of string"] ("location (both)")
        # "Template Separator\n(You can make a copy of, or modify, this frame)"
        n334 = VISA Read(VISA resource name=w1052, byte count=u32 16, error in (no error)=w1050) -> (VISA resource name out=w1051:refnum<visa-resource-name>, read buffer=w1043:string, error out=w1049:errorcluster)  [unwired: 1 out]
        n335 = call <vilib>:"Trim Whitespace.vi"("string"=w1043, "location (both)"=w1042) -> ("trimmed string"=w1041:string)
        n336 = Search/Split String(string=w1041, search string/char (-)="\t") -> (substring before match=w1039:string, match + rest of string=w1038:string)  [unwired: 1 in, 1 out]
        n337 = String Subset(string=w1038, offset (0)=2) -> (substring=w1036:string)  [unwired: 1 in]
        n338 = String Subset(string=w1039, offset (0)=1) -> (substring=w1045:string)  [unwired: 1 in]
        n339 = Hexadecimal String To Number(string=w1036, default (0uL)=u32 0 ("default (0 U32)")) -> (number=w1029:u32)  [unwired: 1 in, 1 out]
        n340 = Hexadecimal String To Number(string=w1045) -> (number=w1033:u32)  [unwired: 2 in, 1 out]
        n341 = Multiply(x=w1033, y=u8 5) -> (x*y=→"CZT 1\nFrequency":u32)
        n342 = Multiply(x=w1029, y=u8 5) -> (x*y=→"CZT 2 \nFrequency":u32)
        n343 = Select(t="", s=w1049, f=w1046) -> (s? t:f=w1047:string)
        n344 = call <vilib>:"Add State(s) to Queue__JKI_lib_State_Machine.vi"("State(s) in Front (\"\")"=w1047, "State(s) in (\"\")"=w1056) -> ("States Out"=w1055:string)  [unwired: 13 in]
      }
      frame "---------- UART Comm ----------" {
        # "UART Communication Separator"
        n345 = call <vilib>:"Add State(s) to Queue__JKI_lib_State_Machine.vi"("State(s) in (\"\")"=w1062) -> ("States Out"=w1061:string)  [unwired: 14 in]
      }
      frame "UART Comm: Init" {
        # "Initialize the UART communication settings"
        n346 = disable-structure shown="Enabled" {
          disable-tunnel: [w1083 T7 {"VISA resource name"="COM7", "baud rate"=115200, "data bits"=8, "parity"=enum."None", "stop bits"=10, "flow control"=0} ("Serial Settings")] -> w1078
          frame Disabled {
            n347 = global read "serialSettings_Global.vi" "Serial Settings"() -> (w1083:T7)
          }
          frame Enabled {
          }
        }
        n348 = Unbundle(w1078) -> ("VISA resource name"=w1077:refnum<visa-resource-name>, "baud rate"=w1076:u32, "data bits"=w1075:u16, "parity"=w1074:enum16{"None", "Odd", "Even", "Mark", "Space"}, "stop bits"=w1073:u16, "flow control"=w1072:u16)
        n349 = call-poly "VISA Configure Serial Port"("VISA resource name"=w1077, "timeout (10sec)"=u32 5000, "termination char\n(0xA = '\\n' = LF)"=u8 10 ("termination char\n(0xA = '\\n' = LF)"), "Enable Termination\nChar (T)"=TRUE ("Enable Termination\nChar (T)"), "baud rate (9600)"=w1076, "data bits (8)"=w1075, "parity (0:none)"=w1074, "error in (no error)"=w1079, "stop bits (10: 1 bit)"=w1073, "flow control (0:none)"=w1072) -> ("VISA resource name out"=w1067:refnum<visa-resource-name>, "error out"=w1066:errorcluster)  [unwired: 4 in]
        n350 = Select(t="", s=w1066, f=w1068) -> (s? t:f=w1071:string)
        n351 = call <vilib>:"Add State(s) to Queue__JKI_lib_State_Machine.vi"("State(s) in Front (\"\")"=w1071, "State(s) in (\"\")"=w1082) -> ("States Out"=w1081:string)  [unwired: 13 in]
      }
      frame "UART Comm: Close" {
        w1091 = T17 128 items=["Flush Receive Buffer"=16, "Write Transmit Buffer to Device"=32, "Flush Receive Buffer (No I/O)"=64, "Flush Transmit Buffer"=128] ("Mask")
        w1090 = T17 16 items=["Flush Receive Buffer"=16, "Write Transmit Buffer to Device"=32, "Flush Receive Buffer (No I/O)"=64, "Flush Transmit Buffer"=128] ("Mask")
        # "Closes the reference to UART"
        n352 = Or(x=w1090, y=w1091) -> (x .or. y?=w1089:T17)
        n353 = VISA Flush I/O Buffer(VISA resource name=w1095, mask (16)=w1089, error in (no error)=w1093) -> (VISA resource name out=w1094:refnum<visa-resource-name>, error out=w1092:errorcluster)
        n354 = VISA Close(VISA resource name=w1094, error in (no error)=w1092) -> (error out=w1087:errorcluster)
        n355 = Select(t="", s=w1087, f=w1086) -> (s? t:f=w1085:string)
        n356 = call <vilib>:"Add State(s) to Queue__JKI_lib_State_Machine.vi"("State(s) in Front (\"\")"=w1085, "State(s) in (\"\")"=w1099) -> ("States Out"=w1098:string)  [unwired: 13 in]
      }
    }
    "States Out" <- w11
  }
  n357 = disable-structure shown="Disabled" {
    frame Disabled {
      n358 = while {
        stop <- _ stop-if-true
        n359 = Get Date/Time In Seconds() -> (seconds since 1Jan1904=→"Current Time":timestamp)
        n360 = Format Date/Time String(time format string (%c)="%m/%d/%Y%H:%M:%S%3u") -> ()  [unwired: 2 in, 1 out]
        n361 = Wait (ms)(milliseconds to wait=u32 1000) -> ()  [unwired: 1 out]
      }
    }
    frame Enabled {
    }
  }
